vi "IR Opo Main.vi"() -> ()   [LabVIEW 2015]
uses:
  System.Windows.Forms
  D:/Fabrizio/Labview Projects/IR OPO Controller/Branches/Final version/uc480DotNet.dll
  uc480DotNet.dll
  <vilib>/Utility/miscctls.llb/LVBoundsTypeDef.ctl
  <vilib>/Utility/config.llb/Read Key (I32).vi
  OPOTEK.dll
  <vilib>/vision/NI_Vision_Development_Module.lvlib
  <vilib>/Utility/config.llb/NI_LVConfig.lvlib
panel:
  in  "Exit 4":bool
  in  "EXIT 3":bool
  in  "EXIT 2":bool
  in  "Laser spot\nX diameter":i32=250
  out "Laser Y offset":string
  out "Laser X offset":string
  in  "Laser offset \nY Position":i32=472 step=1
  in  "Laser offset \nX Position":i32=563 step=1
  out "ROI Rectangle Y position":i32
  out "ROI Rectangle X position":i32
  out "Processi time (sec)":i32
  in  "Processing time unit":string(combo)="sec"
  in  "Mode":i32(ring) items=["RGB 32"=0, "RGB 24"=1, "Y8 Monochrom"=6]
  in  "Camera":refnum<k24>(container)
  in  "Init Camera":bool
  in  "Start Live":bool
  in  "Stop Live":bool
  in  "Load Parameter":bool
  out "Error Out":errorcluster caption="error"
  out "Bits/Pixel":i32=8
  out "Width":i32=8
  out "Height":i32=8
  out "Serial Number":string
  in  "Camera ID":i32
  in  "Zoom":dbl(ring)=1.5 items=["4X"=4.0, "2X"=2.0, "1.5X"=1.5, "1.25X"=1.25, "1X"=1.0]
  in  "Gain Boost":bool=TRUE
  in  "Snapshot":bool
  out "Output":picture
  in  "Exposure":dbl(slide)=33.21525 min=0.06241666666666667 max=99.80425000000001 step=0.06241666666666667 scale=0.06241666666666667..99.80425000000001 scale format="%#.3g"
  in  "Framerate":dbl(slide)=33.21525 min=0.47411700449083627 max=15.001275108384213 step=0.014032998230479876 scale=0.47411700449083627..15.001275108384213 scale format="%#.3g"
  in  "Pixelclock":i32(slide)=33 min=5 max=40 step=1 scale=5.0..40.0
  out "Bits/Pixel 2":i32=8
  out "Width 2":i32=8
  out "Height 2":i32=8
  out "Serial Number 2":string
  in  "error in (no error)":errorcluster
  out "error out":errorcluster
  in  "Y":string="3"
  in  "X":string="2"
  out "# pixels in an ablation spot":i32=625
  in  "Sampling\nPrecision":dbl=0.8 min=0.0 max=1.0 step=0.01 format="%#_13g"
  out "Y step size in pixels":i32=12
  out "Y Step size in µm":i32=120
  out "Commands array":string[][](array[string])
  out "Laser on/off array":bool[][](array[boolean])
  out "Y axis moving time":dbl=250.0
  out "Time array":dbl[][](array[numeric])
  in  "Process Image":bool
  in  "Pixel \nsize":dbl=10.0
  in  "Axes speed \n(µm/s)":i32=500
  in  "Laser spot\nY diameter":i32=250
  in  "Y axis \nprecision":i32=2
  in  "Fast \nsampling?":bool=TRUE
  out "Y size \n(pixels)":i32
  out "X size\n(pixels)":i32
  out "Process time":dbl
  out "X size \n(µm)":i32
  out "Y size \n(µm)":i32
  out "Source":T1(plugin-control)
  in  "Delay":dbl format="%#_13g"
  in  "GPIB Mode":i16
  in  "Open ESP \nManual":bool
  in  "Type a command":string
  in  "Send \nCommand":bool
  out "GPIBtimeout":i32
  out "GPIBtermChar":i32
  out "GPIBport":i32
  out "GPIBdelay":i32
  in  "Run Program":bool
  in  "Capture":bool
  out "Log":string
  in  "Check \nProgram":bool
  out "Laser Operation":bool
  out "Current Wavelength":dbl
  in  "Alignment \ndiode":bool
  in  "LASER":bool
  in  "LAMP":bool
  in  "Wavelength":dbl min=2600.0 max=3200.0 step=1.0
  in  "TUNE":bool
  out "error_Code 3":i32
  in  "Repetition \nRate":enum16{"1", "2", "5", "10", "20"}(ring)=enum."20"
  in  "Energy (%)":i16(slide) min=0 max=100 scale=0.0..100.0 scale format="%#.1f"
  out "error_Code 2":i32
  out "Max":dbl
  out "Min":dbl
  out "error_Code":i32
  out "laserCOMPort":i32
  out "motorCOMPort":i32
  in  "EXIT":bool
  # "Laser Control"
  # "Stages Control"
  # "Camera Control"
  # "ROI Processing"
  # "Axis \nChannels"
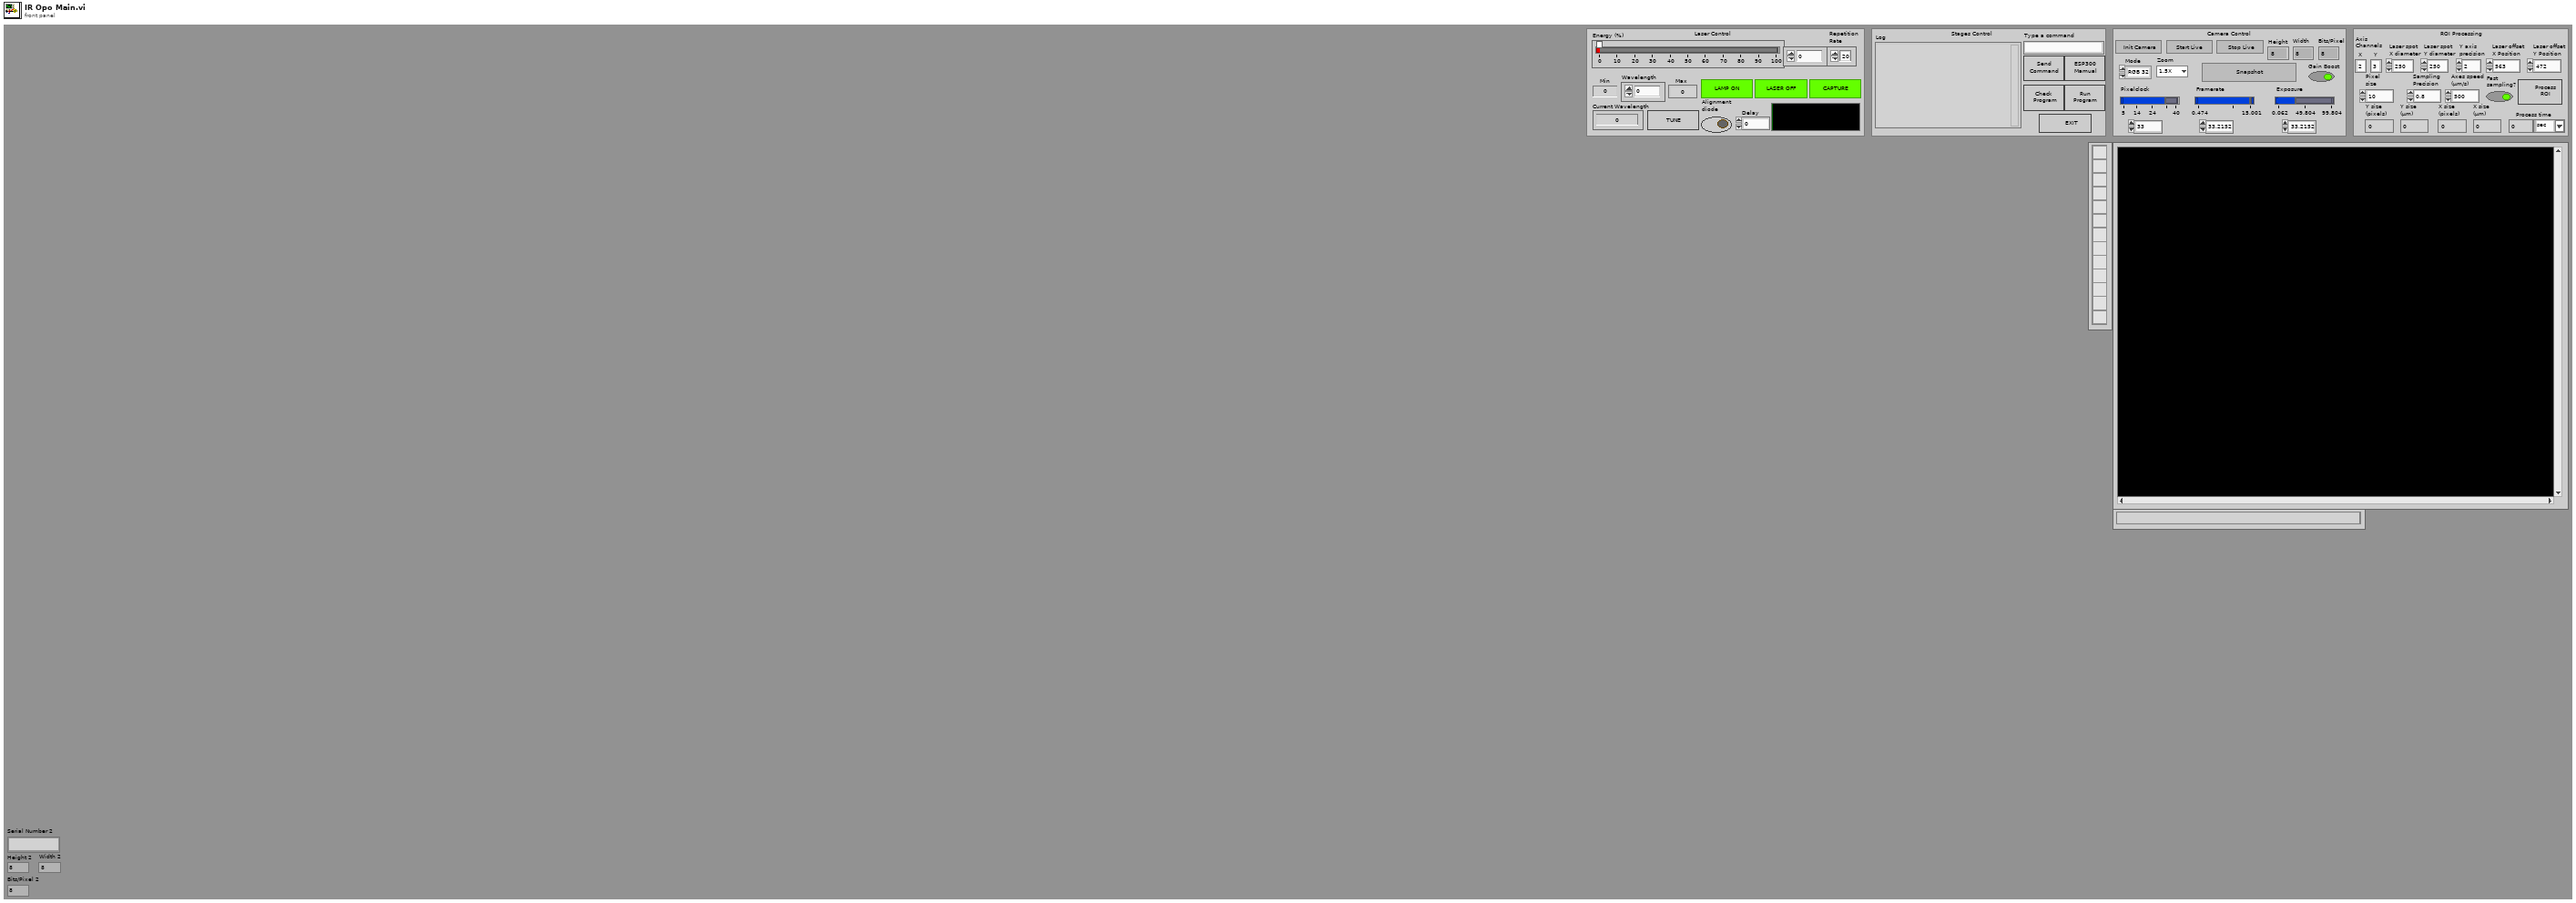
[diagram p1: front panel]
types:
  T1 = typedef "IMAQ Image.ctl" = refnum<image>
  T2 = typedef "LVBoundsTypeDef.ctl" = cluster{"Width":u32, "Height":u32}
  T3 = enum8{"Enabled", "Disabled", "Disabled and Grayed Out"}
  T4 = typedef "NI_LVConfig.lvlib/Config Data RefNum.ctl" = refnum<k1>
  T5 = typedef "Image Type" = u32
  T6 = cluster{"Global Rectangle":i32[], "Contours":cluster{"Contour Type":u32, "ROI Type":u32, "Points":i32[]}[]}
  T7 = enum16{"Initialize", "Lamp ON", "Lamp OFF", "Q-switch ON", "Q-switch OFF", "Adjust Energy", "Change Rep. Rate", "Send String"}
  T8 = enum16{"open", "replace", "create", "open or create", "replace or create", "replace or create with confirmation"}
  T9 = enum32{"invalid app kind", "Development System", "Run Time System", "Student Edition", "Embedded LabVIEW", "Evaluation", "Custom"}
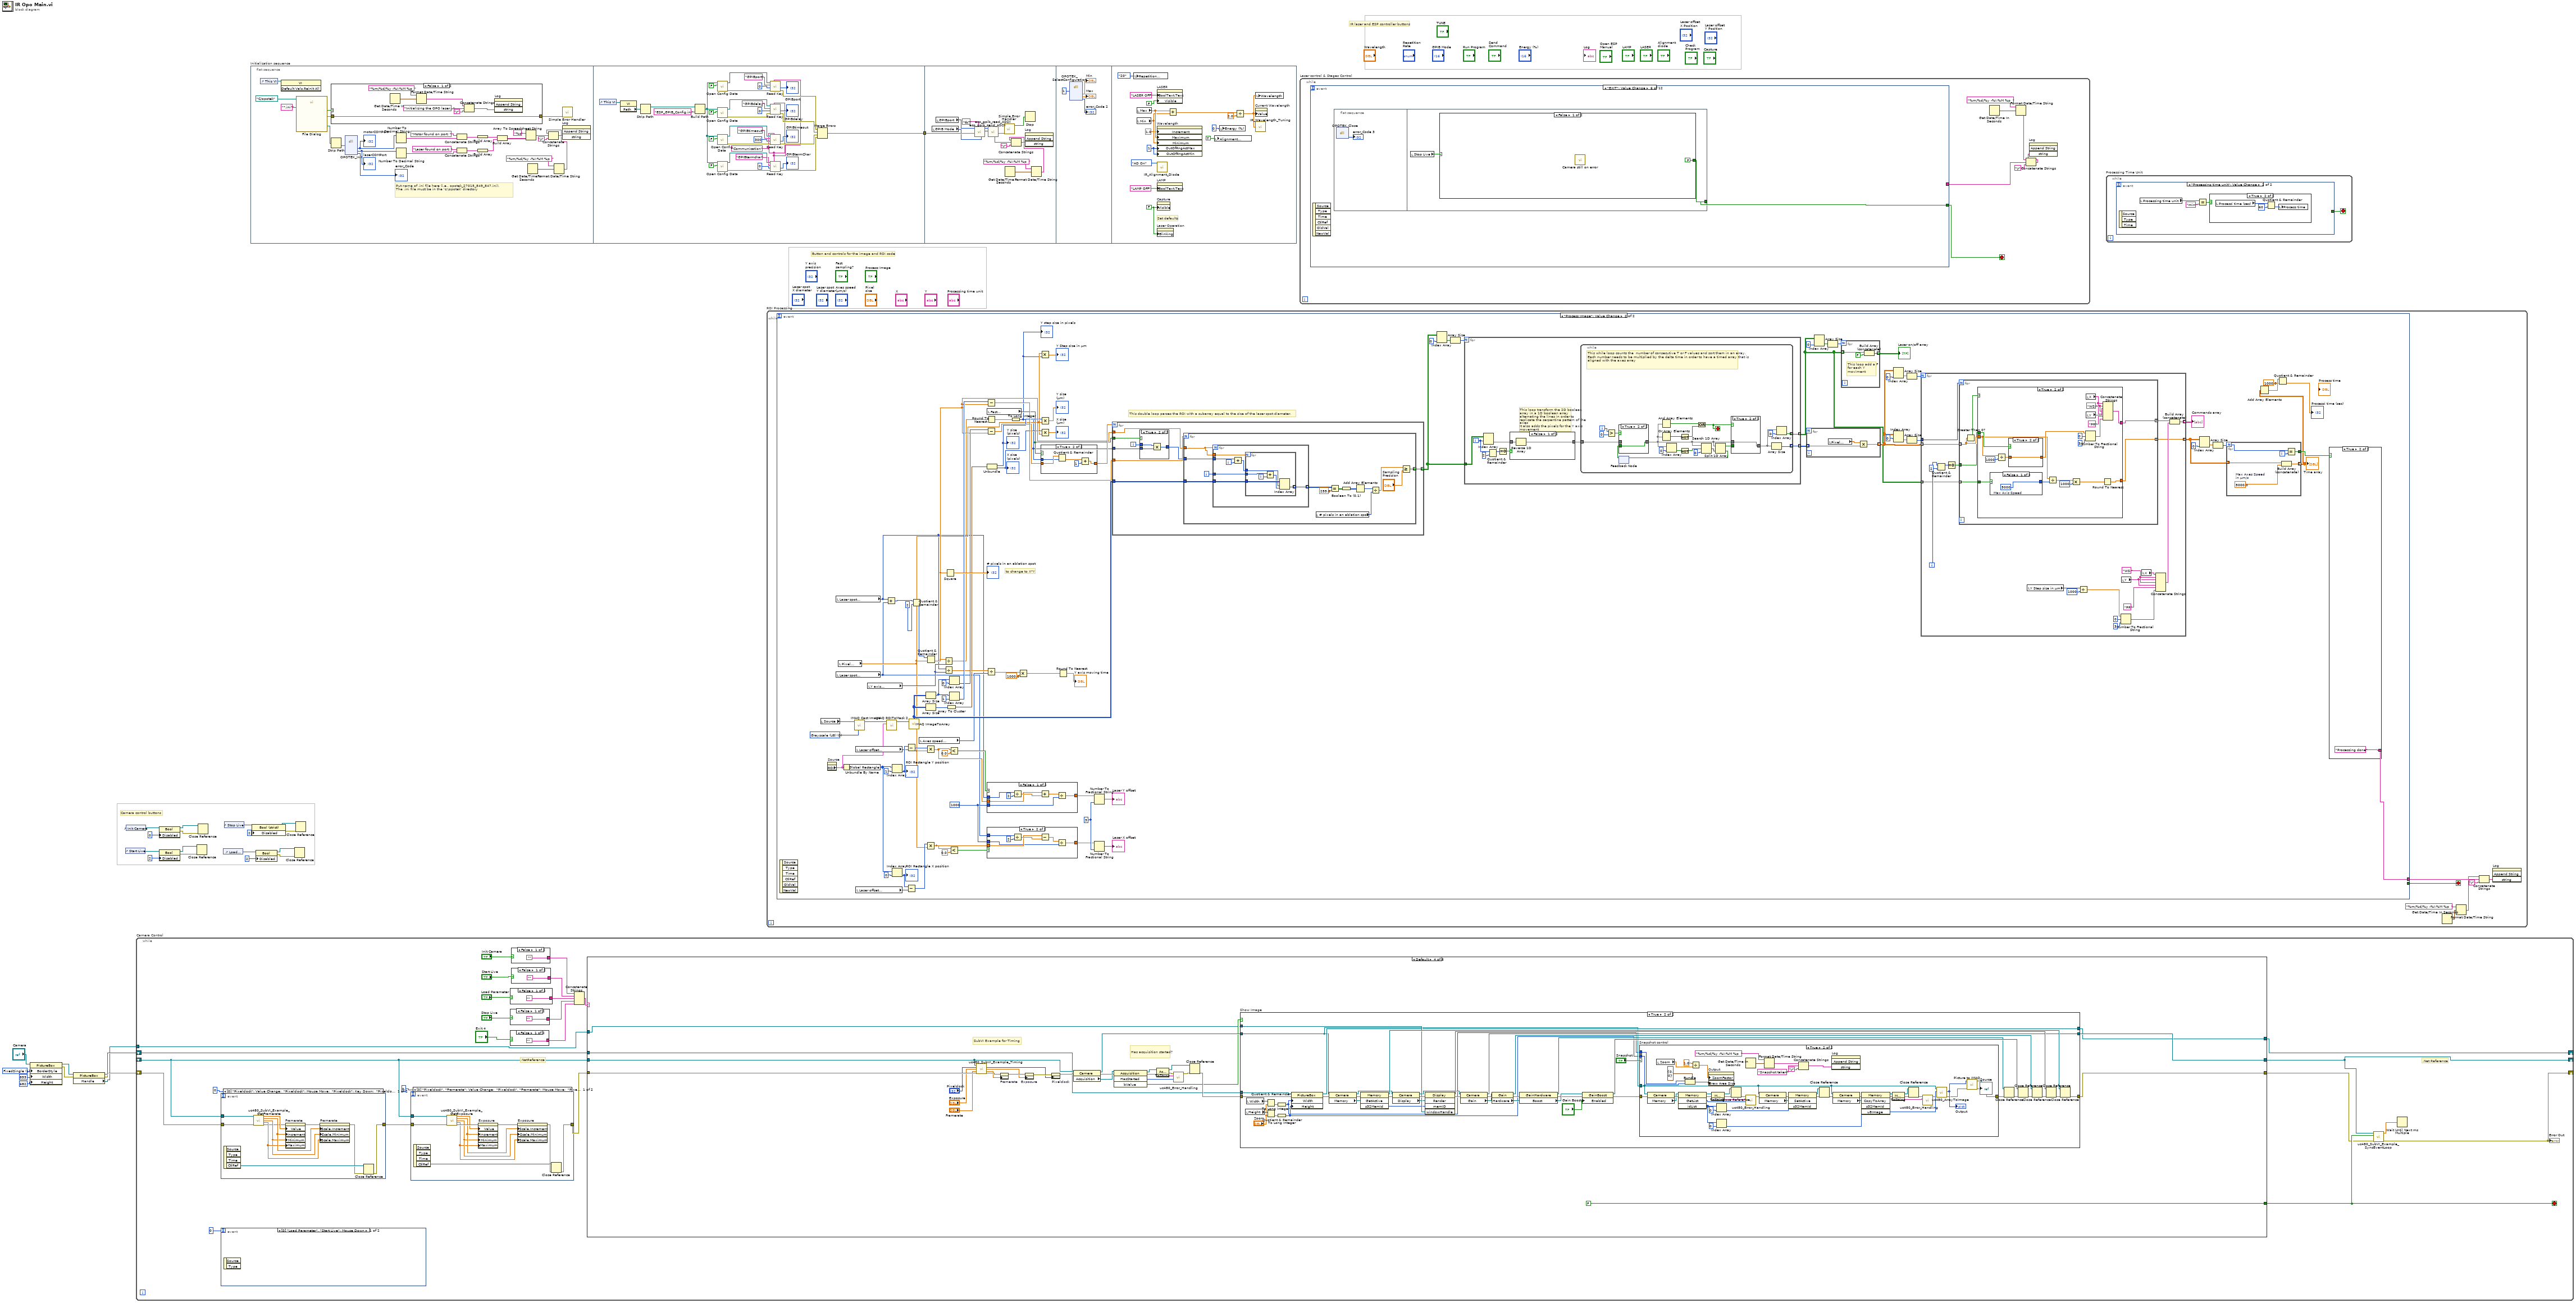
[diagram p0: block diagram]
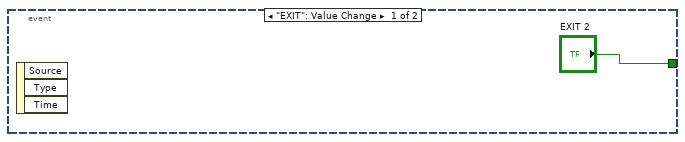
[diagram p2: hidden frame]
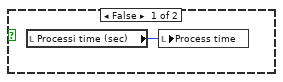
[diagram p3: hidden frame]
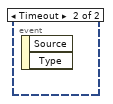
[diagram p4: hidden frame]
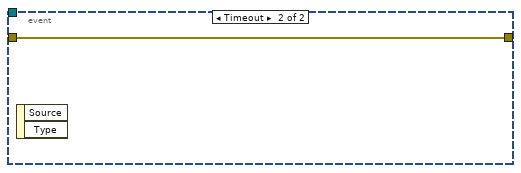
[diagram p5: hidden frame]
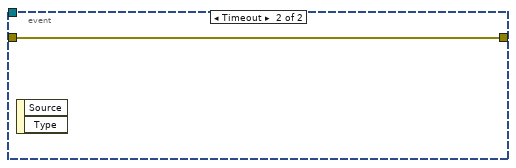
[diagram p6: hidden frame]
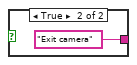
[diagram p7: hidden frame]
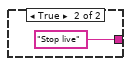
[diagram p8: hidden frame]
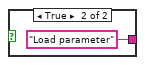
[diagram p9: hidden frame]
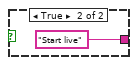
[diagram p10: hidden frame]
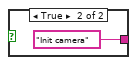
[diagram p11: hidden frame]
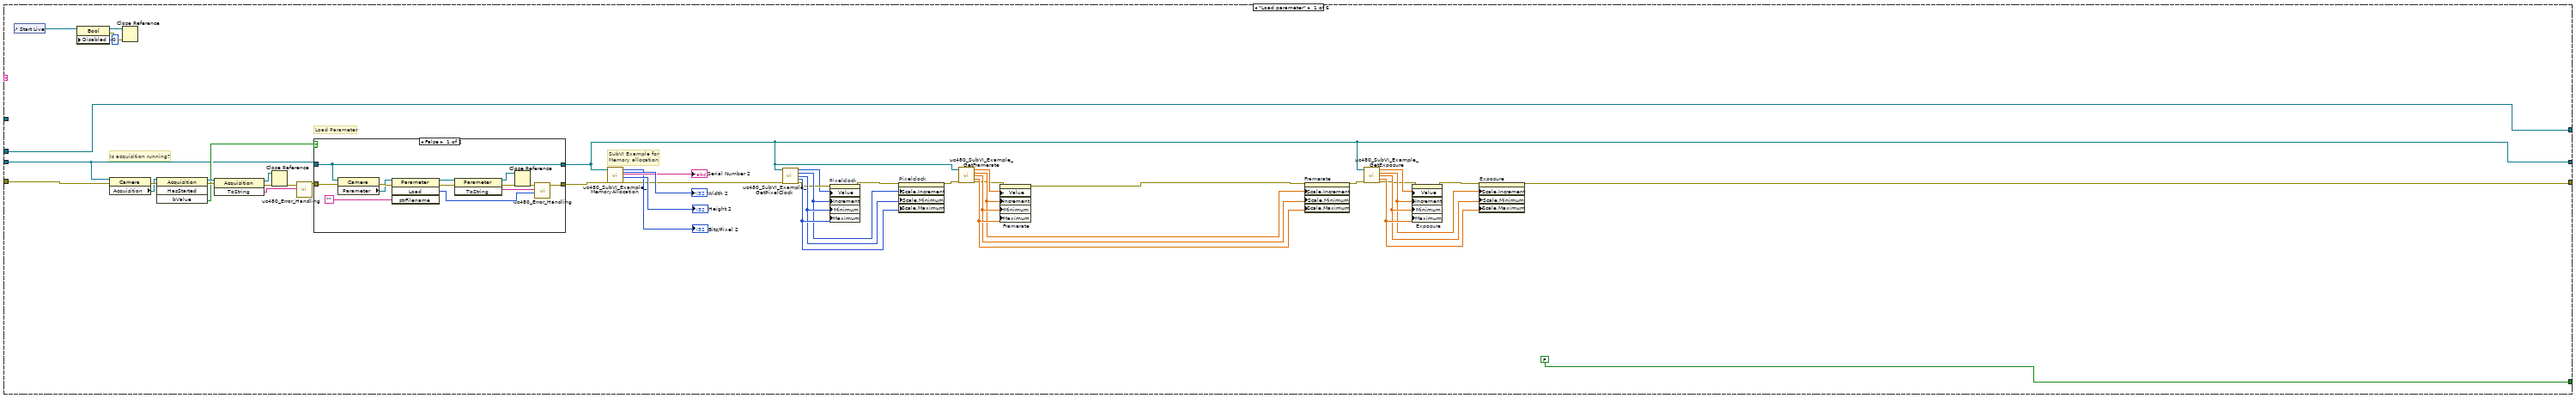
[diagram p12: hidden frame]
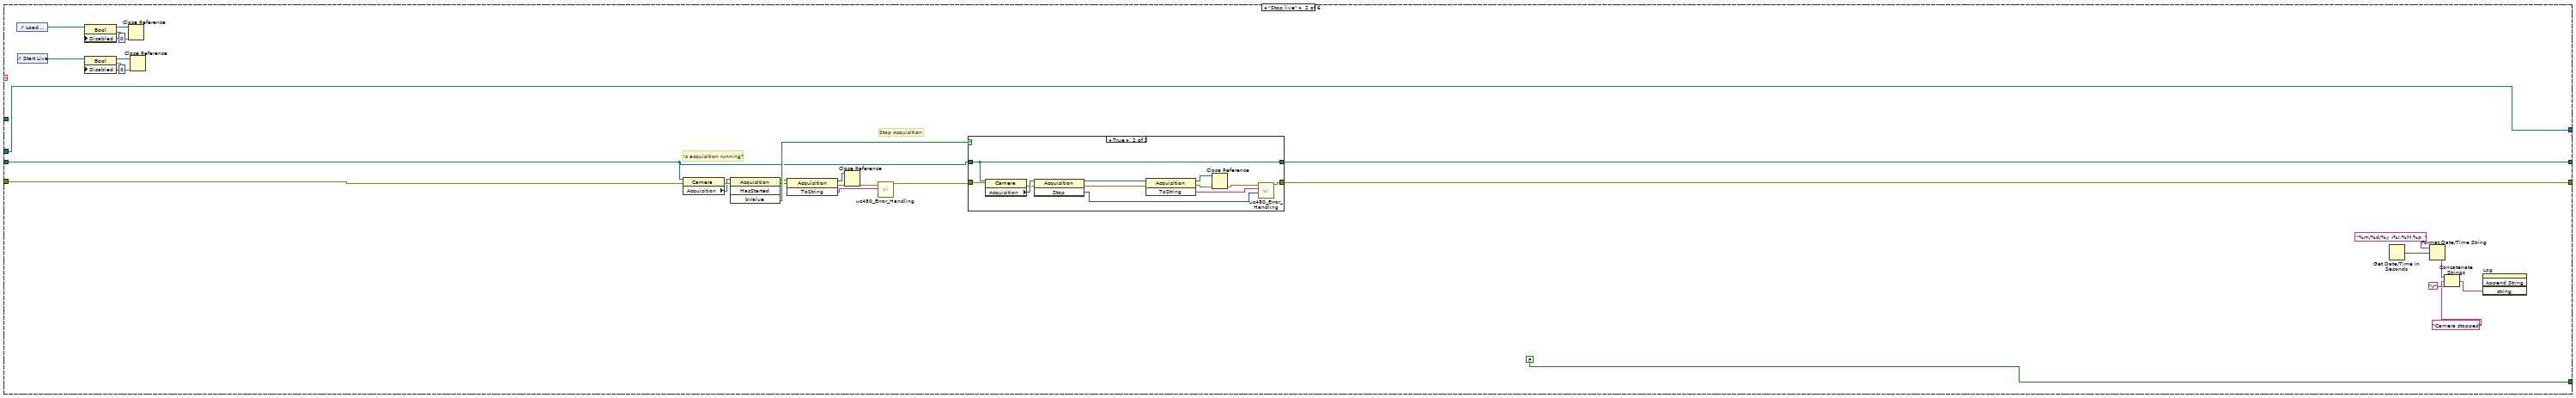
[diagram p14: hidden frame]
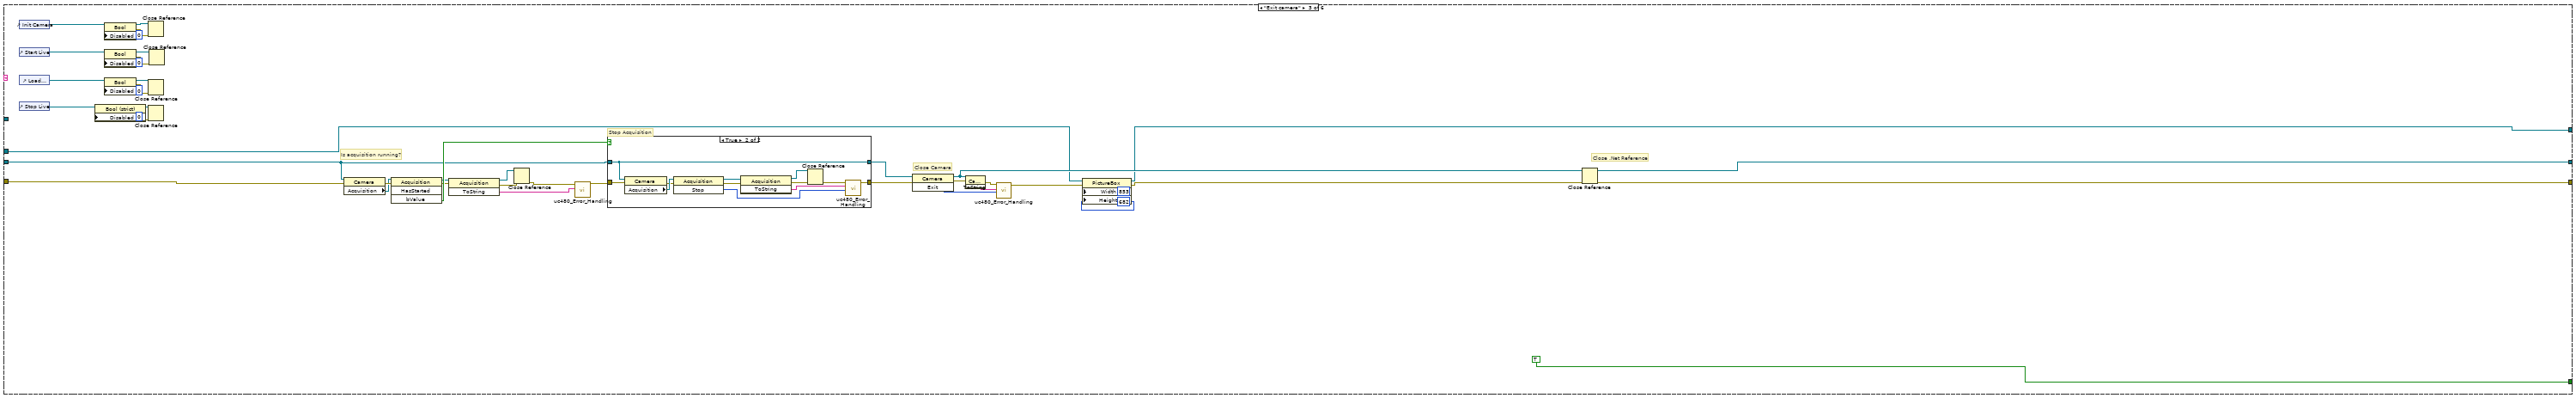
[diagram p16: hidden frame]
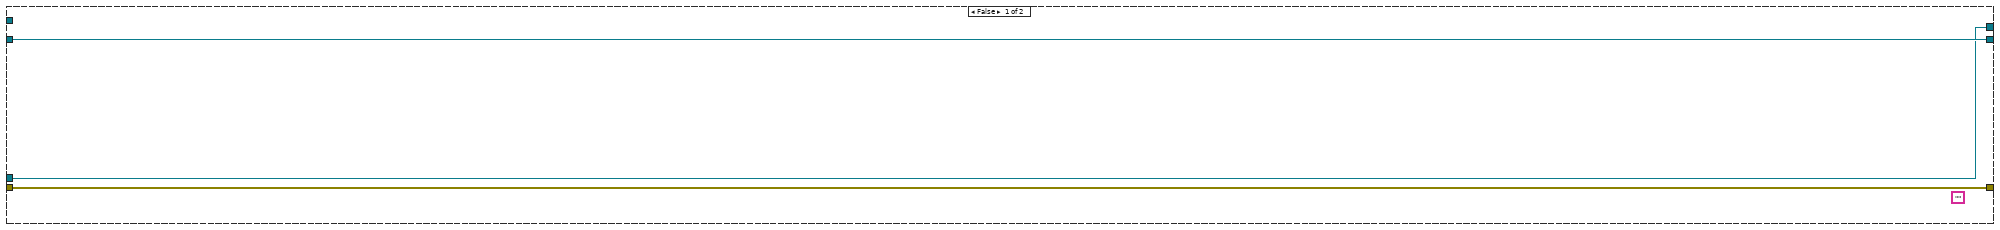
[diagram p18: hidden frame]
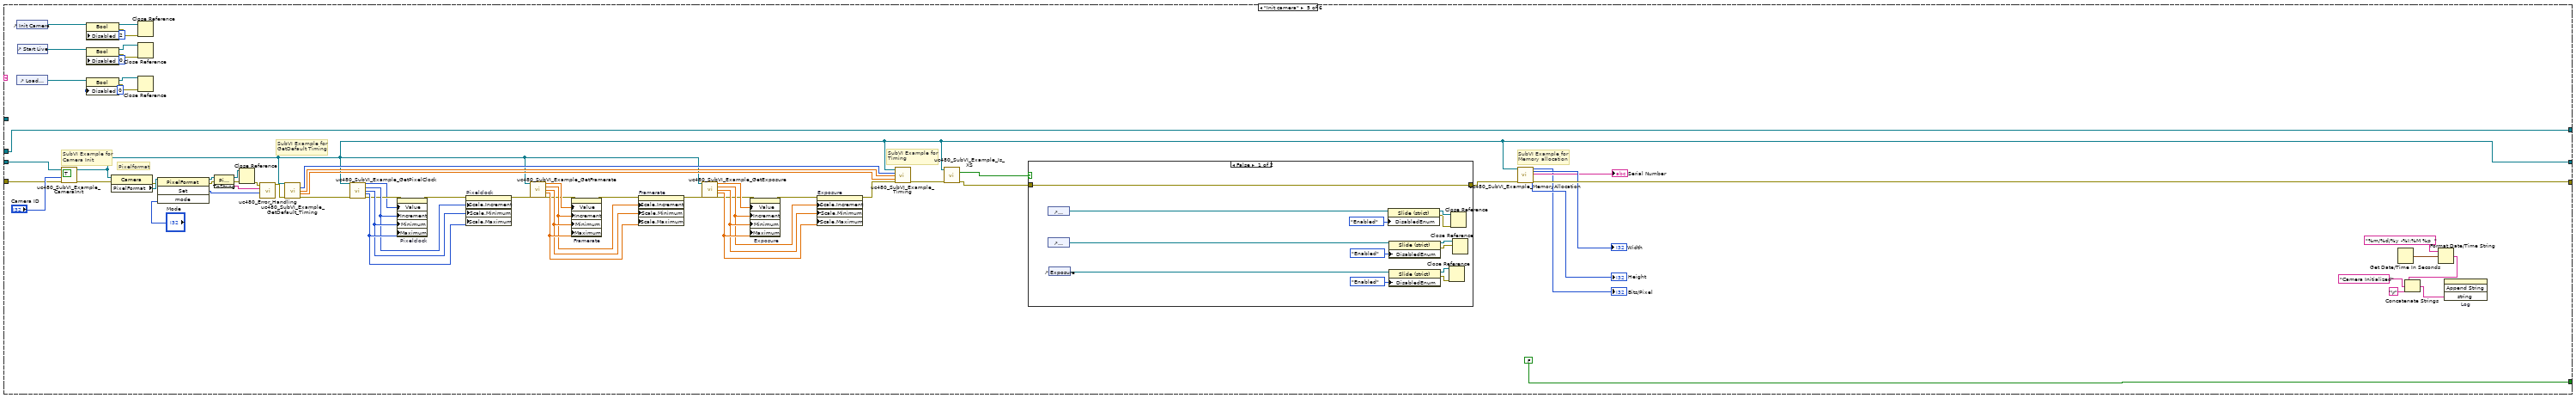
[diagram p20: hidden frame]
diagram:
  w16 = 1 items=["None", "FixedSingle", "Fixed3D"] ("BorderStyle")
  # "Camera control buttons"
  # "IR laser and ESP controller buttons"
  # "Button and controls for the image and ROI code"
  n1 = property class="PictureBox"(reference="Camera", "BorderStyle"=w16, "Width"=853, "Height"=682) -> (reference out=w4:refnum<k24>, error out=w5:errorcluster)  [unwired: 1 in]
  n2 = property class="PictureBox"(reference=w4, error in=w5) -> (reference out=w3:refnum<k24>, error out=w2:errorcluster, "Handle"=w1:refnum<k24>)
  n3 = control-ref of="Start Live"() -> (w22:refnum<vi>)
  n4 = control-ref of="Init Camera"() -> (w25:refnum<vi>)
  n5 = while "Camera Control" {
    shift-right: [w32] -> _
    shift-left: w2 -> [w38]
    shift-right: [w35] -> _
    shift-left: _ -> [w28]
    shift-right: [w30] -> _
    shift-left: w3 -> [w31]
    tunnel: w1 -> [w29]
    stop <- w36 stop-if-true
    # ".NetReference"
    # ".Net Reference"
    n6 = event shown="[0] \"Pixelclock\": Value Change;  \"Pixelclock\": Mouse Move;  \"Pixelclock\": Key Down;  \"Pixelclock\": Mouse Up" {
      selector: _ -> [_ _]
      dyn-events: _ -> [_ _]
      timeout: 0 -> [_ _]
      tunnel: [w53 w64] -> w39
      tunnel: w38 -> [w63 w64]
      tunnel: w28 -> [w62 _]
      event "Pixelclock": Value Change; "Pixelclock": Mouse Move; "Pixelclock": Key Down; "Pixelclock": Mouse Up {
        n7 = event-data() -> ("CtlRef"=w55:refnum<vi>)  [unwired: 1 in, 3 out]
        n8 = call "uc480_SubVI_Example_GetFramerate.vi"(".NET (Reference)"=w62, "Error In"=w63) -> ("Framerate"=w61:dbl, "Inc"=w60:dbl, "Min"=w58:dbl, "Max"=w59:dbl, "error out"=w57:errorcluster)  [unwired: 9 in]
        n9 = property on="Framerate" class="Slide (strict)"(error in=w57, "Value"=w61, "Increment"=w60, "Minimum"=w58, "Maximum"=w59) -> (error out=w56:errorcluster)  [unwired: 1 in, 1 out]
        n10 = property on="Framerate" class="Slide (strict)"(error in=w56, "Scale.Increment"=w60, "Scale.Minimum"=w58, "Scale.Maximum"=w59) -> (error out=w54:errorcluster)  [unwired: 1 in, 1 out]
        n11 = Close Reference(reference=w55, error in (no error)=w54) -> (error out=w53:errorcluster)
      }
      event Timeout {
        n12 = event-data() -> ()  [unwired: 1 in, 2 out]
      }
    }
    n13 = event shown="[0] \"Load Parameter\", \"Start Live\": Mouse Down" {
      selector: _ -> [_ _]
      dyn-events: _ -> [_ _]
      timeout: 0 -> [_ _]
      event "Load Parameter", "Start Live": Mouse Down {
        n14 = event-data() -> ()  [unwired: 1 in, 2 out]
      }
      event Timeout {
        n15 = event-data() -> ()  [unwired: 1 in, 2 out]
      }
    }
    n16 = event shown="[0] \"Pixelclock\", \"Framerate\": Value Change;  \"Pixelclock\", \"Framerate\": Mouse Move;  \"Pixelclock\", \"Framerate\": Key Down;  \"Pixelclock\", \"Framerate\": Mouse Up" {
      selector: _ -> [_ _]
      dyn-events: _ -> [_ _]
      timeout: 0 -> [_ _]
      tunnel: w39 -> [w75 w76]
      tunnel: [w65 w76] -> w41
      tunnel: w28 -> [w74 _]
      event "Pixelclock", "Framerate": Value Change; "Pixelclock", "Framerate": Mouse Move; "Pixelclock", "Framerate": Key Down; "Pixelclock", "Framerate": Mouse Up {
        n17 = event-data() -> ("CtlRef"=w67:refnum<vi>)  [unwired: 1 in, 3 out]
        n18 = call "uc480_SubVI_Example_GetExposure.vi"(".NET (Reference)"=w74, "Error In"=w75) -> ("Exposure"=w71:dbl, "Inc"=w70:dbl, "Min"=w69:dbl, "Max"=w68:dbl, "Error out"=w72:errorcluster)  [unwired: 9 in]
        n19 = property on="Exposure" class="Slide (strict)"(error in=w72, "Value"=w71, "Increment"=w70, "Minimum"=w69, "Maximum"=w68) -> (error out=w73:errorcluster)  [unwired: 1 in, 1 out]
        n20 = property on="Exposure" class="Slide (strict)"(error in=w73, "Scale.Increment"=w70, "Scale.Minimum"=w69, "Scale.Maximum"=w68) -> (error out=w66:errorcluster)  [unwired: 1 in, 1 out]
        n21 = Close Reference(reference=w67, error in (no error)=w66) -> (error out=w65:errorcluster)
      }
      event Timeout {
        n22 = event-data() -> ()  [unwired: 1 in, 2 out]
      }
    }
    n23 = case shown="False" "Exit 4" {
      tunnel: ["" "Exit camera"] -> w43
      frame False {
      }
      frame True {
      }
    }
    n24 = case shown="False" "Load Parameter" {
      tunnel: ["" "Load parameter"] -> w46
      frame False {
      }
      frame True {
      }
    }
    n25 = case shown="False" "Stop Live" {
      tunnel: ["" "Stop live"] -> w45
      frame False {
      }
      frame True {
      }
    }
    n26 = case shown="False" "Init Camera" {
      tunnel: ["" "Init camera"] -> w50
      frame False {
      }
      frame True {
      }
    }
    n27 = case shown="False" "Start Live" {
      tunnel: ["" "Start live"] -> w49
      frame False {
      }
      frame True {
      }
    }
    n28 = Concatenate Strings(w50, w49, w46, w45, w43) -> (w48:string)
    n29 = case shown="Default" w48 {
      tunnel: w28 -> [w123 w169 w219 w261 w437 w494]
      tunnel: w41 -> [w126 w170 w220 w271 w436 w495]
      tunnel: [w93 w168 w228 w270 w395 w493] -> w35
      tunnel: [w94 w167 w229 w269 w432 w491] -> w34
      tunnel: [FALSE FALSE TRUE FALSE FALSE FALSE] -> w36
      tunnel: w31 -> [w92 w161 w201 w253 w390 w484]
      tunnel: [w92 w161 w200 w252 w390 w484] -> w30
      tunnel: w29 -> [_ _ _ w249 _ _]
      frame "Load parameter" {
        # "SubVI Example for \nMemory allocation"
        # "Is acquisition running?"
        # "Load Parameter"
        n30 = control-ref of="Start Live"() -> (w117:refnum<vi>)
        n31 = property class="Bool"(reference=w117, "Disabled"=u8 0 ("Deaktiviert")) -> (reference out=w91:refnum<vi>, error out=w90:errorcluster)  [unwired: 1 in]
        n32 = property class="Camera"(reference=w123, error in=w126) -> (error out=w131:errorcluster, "Acquisition"=w130:refnum<k24>)  [unwired: 1 out]
        n33 = Close Reference(reference=w91, error in (no error)=w90) -> ()  [unwired: 1 out]
        n34 = invoke class="Acquisition" method="HasStarted"(reference=w130, error in=w131) -> (reference out=w127:refnum<k24>, error out=w129:errorcluster, "bValue"=w125:bool)  [unwired: 2 in, 1 out]
        n35 = invoke class="Acquisition" method="ToString"(reference=w127, error in=w129) -> (reference out=w89:refnum<k24>, error out=w88:errorcluster, "ToString"=w128:string)  [unwired: 1 in]
        n36 = Close Reference(reference=w89, error in (no error)=w88) -> (error out=w87:errorcluster)
        n37 = call "uc480_Error_Handling.vi"("Error String"=w128, "Error In"=w87) -> ("Error Out"=w124:errorcluster)  [unwired: 9 in]
        n38 = case shown="False" w125 {
          tunnel: w124 -> [w139 w146]
          tunnel: w123 -> [w137 w147]
          tunnel: [w138 w146] -> w118
          tunnel: [w137 w147] -> w93
          frame False {
            n39 = property class="Camera"(reference=w137, error in=w139) -> (error out=w141:errorcluster, "Parameter"=w140:refnum<k24>)  [unwired: 1 out]
            n40 = invoke class="Parameter" method="Load"(reference=w140, error in=w141, "strFilename"="") -> (reference out=w143:refnum<k24>, error out=w144:errorcluster, "Load"=w136:i32)  [unwired: 1 in, 1 out]
            n41 = invoke class="Parameter" method="ToString"(reference=w143, error in=w144) -> (reference out=w133:refnum<k24>, error out=w135:errorcluster, "ToString"=w145:string)  [unwired: 1 in]
            n42 = Close Reference(reference=w133, error in (no error)=w135) -> (error out=w134:errorcluster)
            n43 = call "uc480_Error_Handling.vi"("Error Code"=w136, "Error String"=w145, "Error In"=w134) -> ("Error Out"=w138:errorcluster)  [unwired: 8 in]
          }
          frame True {
          }
        }
        n44 = call "uc480_SubVI_Example_MemoryAllocation.vi"(".NET (Reference)"=w93, "Error In"=w118) -> ("Bits/Pixel 2"=→"Bits/Pixel 2":i32, "Width"=→"Width 2":i32, "Serial Number"=→"Serial Number 2":string, "Height"=→"Height 2":i32, "Error Out"=w95:errorcluster)  [unwired: 13 in]
        n45 = call "uc480_SubVI_Example_GetPixelClock.vi"(".NET (Reference)"=w93, "Error In"=w95) -> ("Pixel Clock"=w96:i32, "Inc"=w98:i32, "Min"=w99:i32, "Max"=w100:i32, "error out"=w97:errorcluster)  [unwired: 9 in]
        n46 = property on="Pixelclock" class="Slide (strict)"(error in=w97, "Value"=w96, "Increment"=w98, "Minimum"=w99, "Maximum"=w100) -> (error out=w101:errorcluster)  [unwired: 1 in, 1 out]
        n47 = property on="Pixelclock" class="Slide (strict)"(error in=w101, "Scale.Increment"=w98, "Scale.Minimum"=w99, "Scale.Maximum"=w100) -> (error out=w102:errorcluster)  [unwired: 1 in, 1 out]
        n48 = call "uc480_SubVI_Example_GetFramerate.vi"(".NET (Reference)"=w93, "Error In"=w102) -> ("Framerate"=w105:dbl, "Inc"=w106:dbl, "Min"=w107:dbl, "Max"=w108:dbl, "error out"=w104:errorcluster)  [unwired: 9 in]
        n49 = property on="Framerate" class="Slide (strict)"(error in=w104, "Value"=w105, "Increment"=w106, "Minimum"=w107, "Maximum"=w108) -> (error out=w103:errorcluster)  [unwired: 1 in, 1 out]
        n50 = property on="Framerate" class="Slide (strict)"(error in=w103, "Scale.Increment"=w106, "Scale.Minimum"=w107, "Scale.Maximum"=w108) -> (error out=w109:errorcluster)  [unwired: 1 in, 1 out]
        n51 = call "uc480_SubVI_Example_GetExposure.vi"(".NET (Reference)"=w93, "Error In"=w109) -> ("Exposure"=w112:dbl, "Inc"=w113:dbl, "Min"=w114:dbl, "Max"=w115:dbl, "Error out"=w110:errorcluster)  [unwired: 9 in]
        n52 = property on="Exposure" class="Slide (strict)"(error in=w110, "Value"=w112, "Increment"=w113, "Minimum"=w114, "Maximum"=w115) -> (error out=w111:errorcluster)  [unwired: 1 in, 1 out]
        n53 = property on="Exposure" class="Slide (strict)"(error in=w111, "Scale.Increment"=w113, "Scale.Minimum"=w114, "Scale.Maximum"=w115) -> (error out=w94:errorcluster)  [unwired: 1 in, 1 out]
      }
      frame "Stop live" {
        # "Is acquisition running?"
        # "Stop Acquisition"
        n54 = control-ref of="Load Parameter"() -> (w165:refnum<vi>)
        n55 = control-ref of="Start Live"() -> (w162:refnum<vi>)
        n56 = property class="Bool"(reference=w165, "Disabled"=u8 0 ("Deaktiviert")) -> (reference out=w160:refnum<vi>, error out=w159:errorcluster)  [unwired: 1 in]
        n57 = property class="Bool"(reference=w162, "Disabled"=u8 0 ("Deaktiviert")) -> (reference out=w158:refnum<vi>, error out=w157:errorcluster)  [unwired: 1 in]
        n58 = Close Reference(reference=w160, error in (no error)=w159) -> ()  [unwired: 1 out]
        n59 = Close Reference(reference=w158, error in (no error)=w157) -> ()  [unwired: 1 out]
        n60 = property class="Camera"(reference=w169, error in=w170) -> (error out=w177:errorcluster, "Acquisition"=w176:refnum<k24>)  [unwired: 1 out]
        n61 = invoke class="Acquisition" method="HasStarted"(reference=w176, error in=w177) -> (reference out=w171:refnum<k24>, error out=w173:errorcluster, "bValue"=w175:bool)  [unwired: 2 in, 1 out]
        n62 = invoke class="Acquisition" method="ToString"(reference=w171, error in=w173) -> (reference out=w154:refnum<k24>, error out=w156:errorcluster, "ToString"=w172:string)  [unwired: 1 in]
        n63 = Close Reference(reference=w154, error in (no error)=w156) -> (error out=w155:errorcluster)
        n64 = call "uc480_Error_Handling.vi"("Error String"=w172, "Error In"=w155) -> ("Error Out"=w174:errorcluster)  [unwired: 9 in]
        n65 = case shown="True" w175 {
          tunnel: [w179 w190] -> w167
          tunnel: w174 -> [w179 w191]
          tunnel: w169 -> [w178 w183]
          tunnel: [w178 w183] -> w168
          frame False {
          }
          frame True {
            n66 = property class="Camera"(reference=w183, error in=w191) -> (error out=w187:errorcluster, "Acquisition"=w188:refnum<k24>)  [unwired: 1 out]
            n67 = invoke class="Acquisition" method="Stop"(reference=w188, error in=w187) -> (reference out=w185:refnum<k24>, error out=w186:errorcluster, "Stop"=w184:i32)  [unwired: 1 in]
            n68 = invoke class="Acquisition" method="ToString"(reference=w185, error in=w186) -> (reference out=w180:refnum<k24>, error out=w182:errorcluster, "ToString"=w189:string)  [unwired: 1 in]
            n69 = Close Reference(reference=w180, error in (no error)=w182) -> (error out=w181:errorcluster)
            n70 = call "uc480_Error_Handling.vi"("Error Code"=w184, "Error String"=w189, "Error In"=w181) -> ("Error Out"=w190:errorcluster)  [unwired: 8 in]
          }
        }
        n71 = Get Date/Time In Seconds() -> (seconds since 1Jan1904=w149:timestamp)
        n72 = Format Date/Time String(time format string (%c)="%m/%d/%y -%I:%M %p  ", seconds (now)=w149) -> (date/time string=w148:string)  [unwired: 1 in]
        n73 = Concatenate Strings(w148, "Camera stopped", "\r") -> (w153:string)
        n74 = invoke on="Log" class="Str" method="Append String"("string"=w153) -> ()  [unwired: 3 in, 4 out]
      }
      frame "Exit camera" {
        # "Close .Net Reference"
        # "Is acquisition running?"
        # "Stop Acquisition"
        # "Close Camera"
        n75 = control-ref of="Init Camera"() -> (w212:refnum<vi>)
        n76 = control-ref of="Start Live"() -> (w211:refnum<vi>)
        n77 = control-ref of="Load Parameter"() -> (w210:refnum<vi>)
        n78 = control-ref of="Stop Live"() -> (w209:refnum<vi>)
        n79 = property class="Bool (strict)"(reference=w209, "Disabled"=u8 0 ("Deaktiviert")) -> (reference out=w199:refnum<vi>, error out=w198:errorcluster)  [unwired: 1 in]
        n80 = property class="Bool"(reference=w212, "Disabled"=u8 0 ("Deaktiviert")) -> (reference out=w193:refnum<vi>, error out=w192:errorcluster)  [unwired: 1 in]
        n81 = property class="Bool"(reference=w211, "Disabled"=u8 0 ("Deaktiviert")) -> (reference out=w195:refnum<vi>, error out=w194:errorcluster)  [unwired: 1 in]
        n82 = property class="Bool"(reference=w210, "Disabled"=u8 0 ("Deaktiviert")) -> (reference out=w197:refnum<vi>, error out=w196:errorcluster)  [unwired: 1 in]
        n83 = Close Reference(reference=w193, error in (no error)=w192) -> ()  [unwired: 1 out]
        n84 = Close Reference(reference=w197, error in (no error)=w196) -> ()  [unwired: 1 out]
        n85 = Close Reference(reference=w199, error in (no error)=w198) -> ()  [unwired: 1 out]
        n86 = Close Reference(reference=w195, error in (no error)=w194) -> ()  [unwired: 1 out]
        n87 = property class="Camera"(reference=w219, error in=w220) -> (error out=w227:errorcluster, "Acquisition"=w226:refnum<k24>)  [unwired: 1 out]
        n88 = invoke class="Acquisition" method="HasStarted"(reference=w226, error in=w227) -> (reference out=w221:refnum<k24>, error out=w223:errorcluster, "bValue"=w225:bool)  [unwired: 2 in, 1 out]
        n89 = invoke class="Acquisition" method="ToString"(reference=w221, error in=w223) -> (reference out=w206:refnum<k24>, error out=w208:errorcluster, "ToString"=w222:string)  [unwired: 1 in]
        n90 = Close Reference ("Close Referenz")(reference=w206, error in (no error)=w208) -> (error out=w207:errorcluster)
        n91 = call "uc480_Error_Handling.vi"("Error String"=w222, "Error In"=w207) -> ("Error Out"=w224:errorcluster)  [unwired: 9 in]
        n92 = case shown="True" w225 {
          tunnel: [w236 w247] -> w217
          tunnel: w224 -> [w236 w248]
          tunnel: w219 -> [w235 w240]
          tunnel: [w235 w240] -> w218
          frame False {
          }
          frame True {
            n93 = property class="Camera"(reference=w240, error in=w248) -> (error out=w244:errorcluster, "Acquisition"=w245:refnum<k24>)  [unwired: 1 out]
            n94 = invoke class="Acquisition" method="Stop"(reference=w245, error in=w244) -> (reference out=w242:refnum<k24>, error out=w243:errorcluster, "Stop"=w241:i32)  [unwired: 1 in]
            n95 = invoke class="Acquisition" method="ToString"(reference=w242, error in=w243) -> (reference out=w237:refnum<k24>, error out=w239:errorcluster, "ToString"=w246:string)  [unwired: 1 in]
            n96 = Close Reference ("Close Referenz")(reference=w237, error in (no error)=w239) -> (error out=w238:errorcluster)
            n97 = call "uc480_Error_Handling.vi"("Error Code"=w241, "Error String"=w246, "Error In"=w238) -> ("Error Out"=w247:errorcluster)  [unwired: 8 in]
          }
        }
        n98 = invoke class="Camera" method="Exit"(reference=w218, error in=w217) -> (reference out=w228:refnum<k24>, error out=w231:errorcluster, "Exit"=w230:i32)  [unwired: 1 in]
        n99 = invoke class="Camera" method="ToString"(reference=w228, error in=w231) -> (error out=w232:errorcluster, "ToString"=w233:string)  [unwired: 1 in, 1 out]
        n100 = call "uc480_Error_Handling.vi"("Error Code"=w230, "Error String"=w233, "Error In"=w232) -> ("Error Out"=w205:errorcluster)  [unwired: 8 in]
        n101 = property class="PictureBox"(reference=w201, error in=w205, "Width"=853, "Height"=682) -> (reference out=w200:refnum<k24>, error out=w204:errorcluster)
        n102 = Close Reference ("Close Referenz")(reference=w228, error in (no error)=w204) -> (error out=w229:errorcluster)
      }
      frame Default {
        # "SubVI Example for Timing"
        # "Has acquisition started?"
        n103 = call "uc480_SubVI_Example_Timing.vi"(".NET (Reference)"=w261, "Pixelclock"="Pixelclock", "Exposure time"="Exposure", "Framerate"="Framerate", "Error In"=w271) -> ("Pixelclock"=w264:i32, "Exposure time"=w263:dbl, "Framerate"=w262:dbl, "Error Out"=w268:errorcluster)  [unwired: 7 in]
        n104 = property on="Framerate" class="Schieber (strikt)"(error in=w268, "Scale.RngStart"=w262) -> (error out=w267:errorcluster)  [unwired: 1 in, 1 out]
        n105 = property on="Exposure" class="Schieber (strikt)"(error in=w267, "Scale.RngStart"=w263) -> (error out=w266:errorcluster)  [unwired: 1 in, 1 out]
        n106 = property on="Pixelclock" class="Schieber (strikt)"(error in=w266, "Scale.RngStart"=w264) -> (error out=w265:errorcluster)  [unwired: 1 in, 1 out]
        n107 = property class="Camera"(reference=w261, error in=w265) -> (reference out=w254:refnum<k24>, error out=w277:errorcluster, "Acquisition"=w276:refnum<k24>)
        n108 = invoke class="Acquisition" method="HasStarted"(reference=w276, error in=w277) -> (reference out=w251:refnum<k24>, error out=w273:errorcluster, "HasStarted"=w272:i32, "bValue"=w250:bool)  [unwired: 2 in]
        n109 = invoke class="Acquisition" method="ToString"(reference=w251, error in=w273) -> (reference out=w255:refnum<k24>, error out=w275:errorcluster, "ToString"=w274:string)  [unwired: 1 in]
        n110 = call "uc480_Error_Handling.vi"("Error Code"=w272, "Error String"=w274, "Error In"=w275) -> ("Error Out"=w257:errorcluster)  [unwired: 8 in]
        n111 = Close Reference(reference=w255, error in (no error)=w257) -> (error out=w256:errorcluster)
        n112 = case "Show Image" shown="True" w250 {
          tunnel: [w281 w293] -> w269
          tunnel: w256 -> [w281 w321]
          tunnel: w254 -> [w280 w285]
          tunnel: [w280 w289] -> w270
          tunnel: w253 -> [w279 w310]
          tunnel: [w279 w287] -> w252
          tunnel: w249 -> [_ w317]
          frame False {
            (unwired) ""
          }
          frame True {
            n113 = local read "Height"() -> (w314:i32)
            n114 = local read "Width"() -> (w315:i32)
            n115 = Quotient & Remainder(x=w315, y="Zoom") -> (floor(x/y)=w312:dbl)  [unwired: 1 out]
            n116 = Quotient & Remainder(x=w314, y="Zoom") -> (floor(x/y)=w311:dbl)  [unwired: 1 out]
            n117 = To Long Integer(number=w312) -> (32bit integer=w284:i32)
            n118 = To Long Integer(number=w311) -> (32bit integer=w283:i32)
            n119 = property class="PictureBox"(reference=w310, error in=w321, "Width"=w284, "Height"=w283) -> (reference out=w287:refnum<k24>, error out=w316:errorcluster)
            n120 = property class="Camera"(reference=w285, error in=w316) -> (reference out=w286:refnum<k24>, error out=w323:errorcluster, "Memory"=w324:refnum<k24>)
            n121 = invoke class="Memory" method="GetActive"(reference=w324, error in=w323) -> (reference out=w318:refnum<k24>, error out=w319:errorcluster, "s32MemId"=w290:i32)  [unwired: 2 in, 1 out]
            n122 = property class="Camera"(reference=w286, error in=w319) -> (reference out=w298:refnum<k24>, error out=w322:errorcluster, "Display"=w307:refnum<k24>)
            n123 = invoke class="Display" method="Render"(reference=w307, error in=w322, "memID"=w290, "windowHandle"=w317) -> (reference out=w308:refnum<k24>, error out=w309:errorcluster)  [unwired: 1 in, 3 out]
            n124 = property class="Camera"(reference=w298, error in=w309) -> (reference out=w289:refnum<k24>, error out=w305:errorcluster, "Gain"=w303:refnum<k24>)
            n125 = property class="Gain"(reference=w303, error in=w305) -> (reference out=w304:refnum<k24>, error out=w300:errorcluster, "Hardware"=w299:refnum<k24>)
            n126 = property class="GainHardware"(reference=w299, error in=w300) -> (reference out=w296:refnum<k24>, error out=w301:errorcluster, "Boost"=w302:refnum<k24>)
            n127 = property class="GainBoost"(reference=w302, error in=w301, "Enabled"="Gain Boost") -> (reference out=w297:refnum<k24>, error out=w288:errorcluster)
            n128 = case "Snapshot control" shown="True" "Snapshot" {
              tunnel: w285 -> [_ w343]
              tunnel: w288 -> [w325 w347]
              tunnel: [w325 w334] -> w282
              tunnel: w284 -> [_ w337]
              tunnel: w283 -> [_ w336]
              frame False {
              }
              frame True {
                n129 = property class="Camera"(reference=w343, error in=w347) -> (error out=w367:errorcluster, "Memory"=w366:refnum<k24>)  [unwired: 1 out]
                n130 = local read "Zoom"() -> (w342:dbl)
                n131 = invoke class="Memory" method="GetList"(reference=w366, error in=w367) -> (reference out=w372:refnum<k24>, error out=w371:errorcluster, "GetList"=w373:i32, "idList"=w360:i32[])  [unwired: 2 in]
                n132 = Bundle(cluster=T2 {"Width"=0, "Height"=0} ("Draw Area Size"), "Width"=w337, "Height"=w336) -> (w338:T2)
                n133 = Divide(x=1.0, y=w342) -> (x/y=w340:dbl)
                n134 = property on="Output" class="Pict"("ZoomFactor"=w340, "Draw Area Size"=w338) -> ()  [unwired: 2 in, 2 out]
                n135 = invoke class="Memory" method="ToString"(reference=w372, error in=w371) -> (reference out=w345:refnum<k24>, error out=w355:errorcluster, "ToString"=w370:string)  [unwired: 1 in]
                n136 = Index Array(array=w360, index=0 ("Active \nAcquisition Buffer")) -> (element=w357:i32)
                n137 = Index Array(array=w360, index=u32 0 ("Active \nOutput Buffer")) -> (element=w356:i32)
                n138 = Close Reference(reference=w345, error in (no error)=w355) -> (error out=w354:errorcluster)
                n139 = Get Date/Time In Seconds() -> (seconds since 1Jan1904=w327:timestamp)
                n140 = call "uc480_Error_Handling.vi"("Error Code"=w373, "Error String"=w370, "Error In"=w354) -> ("Error Out"=w363:errorcluster)  [unwired: 8 in]
                n141 = property class="Camera"(reference=w343, error in=w363) -> (error out=w362:errorcluster, "Memory"=w361:refnum<k24>)  [unwired: 1 out]
                n142 = Format Date/Time String(time format string (%c)="%m/%d/%y -%I:%M %p  ", seconds (now)=w327) -> (date/time string=w326:string)  [unwired: 1 in]
                n143 = invoke class="Memory" method="SetActive"(reference=w361, error in=w362, "s32MemId"=w357) -> (reference out=w346:refnum<k24>, error out=w353:errorcluster)  [unwired: 1 in, 2 out]
                n144 = Concatenate Strings(w326, "Snapshot taken", "\r") -> (w331:string)
                n145 = Close Reference(reference=w346, error in (no error)=w353) -> (error out=w352:errorcluster)
                n146 = invoke on="Log" class="Str" method="Append String"("string"=w331) -> ()  [unwired: 3 in, 4 out]
                n147 = property class="Camera"(reference=w343, error in=w352) -> (error out=w369:errorcluster, "Memory"=w358:refnum<k24>)  [unwired: 1 out]
                n148 = invoke class="Memory" method="CopyToArray"(reference=w358, error in=w369, "s32MemId"=w356) -> (reference out=w348:refnum<k24>, error out=w349:errorcluster, "u8Image"=w368:u8[])  [unwired: 2 in, 2 out]
                n149 = invoke class="Memory" method="ToString"(reference=w348, error in=w349) -> (reference out=w344:refnum<k24>, error out=w351:errorcluster, "ToString"=w374:string)  [unwired: 1 in]
                n150 = Close Reference(reference=w344, error in (no error)=w351) -> (error out=w350:errorcluster)
                n151 = call "uc480_Error_Handling.vi"("Error String"=w374, "Error In"=w350) -> ("Error Out"=w365:errorcluster)  [unwired: 9 in]
                n152 = call "uc480_ArrayToImage.vi"("Error In"=w365, "InArray"=w368, ".NET (Reference)"=w343) -> ("Error Out"=w333:errorcluster, "Image"=w335:picture)  [unwired: 7 in]
                "Output" <- w335
                n153 = call "Picture to IMAQ.vi"("Error In"=w333, "picture"=w335) -> ("Error Out"=w334:errorcluster, "Image"=→"Source":T1)  [unwired: 8 in]
              }
            }
            n154 = Close Reference(reference=w296, error in (no error)=w282) -> (error out=w295:errorcluster)
            n155 = Close Reference(reference=w297, error in (no error)=w295) -> (error out=w292:errorcluster)
            n156 = Close Reference(reference=w304, error in (no error)=w292) -> (error out=w306:errorcluster)
            n157 = Close Reference(reference=w308, error in (no error)=w306) -> (error out=w320:errorcluster)
            n158 = Close Reference(reference=w318, error in (no error)=w320) -> (error out=w293:errorcluster)
          }
        }
      }
      frame "Init camera" {
        # "SubVI Example for \nGetDefault Timing"
        # "SubVI Example for \nMemory allocation"
        # "SubVI Example for \nTiming"
        # "SubVI Example for \nCamera Init"
        # "Pixelformat"
        n159 = control-ref of="Init Camera"() -> (w400:refnum<vi>)
        n160 = control-ref of="Load Parameter"() -> (w396:refnum<vi>)
        n161 = control-ref of="Start Live"() -> (w398:refnum<vi>)
        n162 = call "uc480_SubVI_Example_CameraInit.vi"("Error In"=w436, "Camera ID"="Camera ID", "Init Camera Flag"=TRUE, ".NET (Reference)"=w437) -> ("Error Out"=w442:errorcluster, ".NET (Reference)"=w395:refnum<k24>)  [unwired: 6 in]
        n163 = property class="Bool"(reference=w396, "Disabled"=u8 0 ("Deaktiviert")) -> (reference out=w385:refnum<vi>, error out=w384:errorcluster)  [unwired: 1 in]
        n164 = property class="Bool"(reference=w400, "Disabled"=u8 2 ("Deaktiviert")) -> (reference out=w389:refnum<vi>, error out=w388:errorcluster)  [unwired: 1 in]
        n165 = property class="Bool"(reference=w398, "Disabled"=u8 0 ("Deaktiviert")) -> (reference out=w387:refnum<vi>, error out=w386:errorcluster)  [unwired: 1 in]
        n166 = property on="Property Node" class="Camera"(reference=w395, error in=w442) -> (error out=w443:errorcluster, "PixelFormat"=w444:refnum<k24>)  [unwired: 1 out]
        n167 = Close Reference(reference=w389, error in (no error)=w388) -> ()  [unwired: 1 out]
        n168 = Close Reference(reference=w387, error in (no error)=w386) -> ()  [unwired: 1 out]
        n169 = Close Reference(reference=w385, error in (no error)=w384) -> ()  [unwired: 1 out]
        n170 = invoke class="PixelFormat" method="Set"(reference=w444, error in=w443, "mode"="Mode") -> (reference out=w440:refnum<k24>, error out=w433:errorcluster, "Set"=w439:i32)  [unwired: 1 in, 1 out]
        n171 = invoke class="PixelFormat" method="ToString"(reference=w440, error in=w433) -> (reference out=w381:refnum<k24>, error out=w383:errorcluster, "ToString"=w441:string)  [unwired: 1 in]
        n172 = Close Reference(reference=w381, error in (no error)=w383) -> (error out=w382:errorcluster)
        n173 = call "uc480_Error_Handling.vi"("Error Code"=w439, "Error String"=w441, "Error In"=w382) -> ("Error Out"=w407:errorcluster)  [unwired: 8 in]
        n174 = call "uc480_SubVI_Example_GetDefault_Timing.vi"(".NET (Reference)"=w395, "Error In"=w407) -> ("Pixelclock"=w406:i32, "Exposure time"=w405:dbl, "Framerate"=w404:dbl, "Error Out"=w403:errorcluster)  [unwired: 10 in]
        n175 = call "uc480_SubVI_Example_GetPixelClock.vi"(".NET (Reference)"=w395, "Error In"=w403) -> ("Pixel Clock"=w408:i32, "Inc"=w410:i32, "Min"=w411:i32, "Max"=w412:i32, "error out"=w409:errorcluster)  [unwired: 9 in]
        n176 = property on="Pixelclock" class="Slide (strict)"(error in=w409, "Value"=w408, "Increment"=w410, "Minimum"=w411, "Maximum"=w412) -> (error out=w413:errorcluster)  [unwired: 1 in, 1 out]
        n177 = property on="Pixelclock" class="Slide (strict)"(error in=w413, "Scale.Increment"=w410, "Scale.Minimum"=w411, "Scale.Maximum"=w412) -> (error out=w414:errorcluster)  [unwired: 1 in, 1 out]
        n178 = call "uc480_SubVI_Example_GetFramerate.vi"(".NET (Reference)"=w395, "Error In"=w414) -> ("Framerate"=w417:dbl, "Inc"=w418:dbl, "Min"=w419:dbl, "Max"=w420:dbl, "error out"=w416:errorcluster)  [unwired: 9 in]
        n179 = property on="Framerate" class="Slide (strict)"(error in=w416, "Value"=w417, "Increment"=w418, "Minimum"=w419, "Maximum"=w420) -> (error out=w415:errorcluster)  [unwired: 1 in, 1 out]
        n180 = property on="Framerate" class="Slide (strict)"(error in=w415, "Scale.Increment"=w418, "Scale.Minimum"=w419, "Scale.Maximum"=w420) -> (error out=w421:errorcluster)  [unwired: 1 in, 1 out]
        n181 = call "uc480_SubVI_Example_GetExposure.vi"(".NET (Reference)"=w395, "Error In"=w421) -> ("Exposure"=w424:dbl, "Inc"=w425:dbl, "Min"=w426:dbl, "Max"=w427:dbl, "Error out"=w422:errorcluster)  [unwired: 9 in]
        n182 = property on="Exposure" class="Slide (strict)"(error in=w422, "Value"=w424, "Increment"=w425, "Minimum"=w426, "Maximum"=w427) -> (error out=w423:errorcluster)  [unwired: 1 in, 1 out]
        n183 = property on="Exposure" class="Slide (strict)"(error in=w423, "Scale.Increment"=w425, "Scale.Minimum"=w426, "Scale.Maximum"=w427) -> (error out=w402:errorcluster)  [unwired: 1 in, 1 out]
        n184 = call "uc480_SubVI_Example_Timing.vi"(".NET (Reference)"=w395, "Pixelclock"=w406, "Exposure time"=w405, "Framerate"=w404, "Error In"=w402) -> ("Error Out"=w394:errorcluster)  [unwired: 7 in, 3 out]
        n185 = call "uc480_SubVI_Example_Is_XS.vi"("Error In"=w394, ".NET (Reference)"=w395) -> ("Error Out"=w391:errorcluster, "IsXS"=w393:bool)  [unwired: 7 in, 1 out]
        n186 = case shown="False" w393 {
          tunnel: w391 -> [w458 w471]
          tunnel: [w458 w471] -> w392
          frame False {
            n187 = control-ref of="Pixelclock"() -> (w454:refnum<vi>)
            n188 = control-ref of="Framerate"() -> (w453:refnum<vi>)
            n189 = control-ref of="Exposure"() -> (w452:refnum<vi>)
            n190 = property class="Slide (strict)"(reference=w454, "DisabledEnum"=T3."Enabled" ("Disabled")) -> (reference out=w451:refnum<vi>, error out=w450:errorcluster)  [unwired: 1 in]
            n191 = property class="Slide (strict)"(reference=w453, "DisabledEnum"=T3."Enabled" ("Disabled")) -> (reference out=w449:refnum<vi>, error out=w448:errorcluster)  [unwired: 1 in]
            n192 = property class="Slide (strict)"(reference=w452, "DisabledEnum"=T3."Enabled" ("Disabled")) -> (reference out=w447:refnum<vi>, error out=w446:errorcluster)  [unwired: 1 in]
            n193 = Close Reference(reference=w447, error in (no error)=w446) -> ()  [unwired: 1 out]
            n194 = Close Reference(reference=w451, error in (no error)=w450) -> ()  [unwired: 1 out]
            n195 = Close Reference(reference=w449, error in (no error)=w448) -> ()  [unwired: 1 out]
          }
          frame True {
            n196 = control-ref of="Pixelclock"() -> (w470:refnum<vi>)
            n197 = control-ref of="Framerate"() -> (w467:refnum<vi>)
            n198 = control-ref of="Exposure"() -> (w465:refnum<vi>)
            n199 = property class="Slide (strict)"(reference=w470, "DisabledEnum"=T3."Disabled and Grayed Out" ("Disabled")) -> (reference out=w463:refnum<vi>, error out=w464:errorcluster)  [unwired: 1 in]
            n200 = property class="Slide (strict)"(reference=w467, "DisabledEnum"=T3."Disabled and Grayed Out" ("Disabled")) -> (reference out=w462:refnum<vi>, error out=w461:errorcluster)  [unwired: 1 in]
            n201 = property class="Slide (strict)"(reference=w465, "DisabledEnum"=T3."Disabled and Grayed Out" ("Disabled")) -> (reference out=w460:refnum<vi>, error out=w459:errorcluster)  [unwired: 1 in]
            n202 = Close Reference(reference=w462, error in (no error)=w461) -> ()  [unwired: 1 out]
            n203 = Close Reference(reference=w460, error in (no error)=w459) -> ()  [unwired: 1 out]
            n204 = Close Reference(reference=w463, error in (no error)=w464) -> ()  [unwired: 1 out]
          }
        }
        n205 = call "uc480_SubVI_Example_MemoryAllocation.vi"(".NET (Reference)"=w395, "Error In"=w392) -> ("Bits/Pixel 2"=→"Bits/Pixel":i32, "Width"=→"Width":i32, "Serial Number"=→"Serial Number":string, "Height"=→"Height":i32, "Error Out"=w432:errorcluster)  [unwired: 13 in]
        n206 = Get Date/Time In Seconds() -> (seconds since 1Jan1904=w376:timestamp)
        n207 = Format Date/Time String(time format string (%c)="%m/%d/%y -%I:%M %p  ", seconds (now)=w376) -> (date/time string=w375:string)  [unwired: 1 in]
        n208 = Concatenate Strings(w375, "Camera Initialized", "\r") -> (w380:string)
        n209 = invoke on="Log" class="Str" method="Append String"("string"=w380) -> ()  [unwired: 3 in, 4 out]
      }
      frame "Start live" {
        # "Has acquisition started?"
        # "Start Acquisition"
        n210 = control-ref of="Start Live"() -> (w490:refnum<vi>)
        n211 = control-ref of="Load Parameter"() -> (w487:refnum<vi>)
        n212 = control-ref of="Stop Live"() -> (w485:refnum<vi>)
        n213 = property class="Bool (strict)"(reference=w485, "Disabled"=u8 0 ("Deaktiviert")) -> (reference out=w483:refnum<vi>, error out=w482:errorcluster)  [unwired: 1 in]
        n214 = property class="Bool"(reference=w490, "Disabled"=u8 2 ("Deaktiviert")) -> (reference out=w479:refnum<vi>, error out=w478:errorcluster)  [unwired: 1 in]
        n215 = property class="Bool"(reference=w487, "Disabled"=u8 2 ("Deaktiviert")) -> (reference out=w481:refnum<vi>, error out=w480:errorcluster)  [unwired: 1 in]
        n216 = Close Reference(reference=w481, error in (no error)=w480) -> ()  [unwired: 1 out]
        n217 = Close Reference(reference=w479, error in (no error)=w478) -> ()  [unwired: 1 out]
        n218 = Close Reference(reference=w483, error in (no error)=w482) -> ()  [unwired: 1 out]
        n219 = property class="Camera"(reference=w494, error in=w495) -> (error out=w504:errorcluster, "Acquisition"=w503:refnum<k24>)  [unwired: 1 out]
        n220 = invoke class="Acquisition" method="HasStarted"(reference=w503, error in=w504) -> (reference out=w499:refnum<k24>, error out=w498:errorcluster, "HasStarted"=w497:i32, "bValue"=w502:bool)  [unwired: 2 in]
        n221 = invoke class="Acquisition" method="ToString"(reference=w499, error in=w498) -> (error out=w501:errorcluster, "ToString"=w500:string)  [unwired: 1 in, 1 out]
        n222 = call "uc480_Error_Handling.vi"("Error Code"=w497, "Error String"=w500, "Error In"=w501) -> ("Error Out"=w496:errorcluster)  [unwired: 8 in]
        n223 = case shown="False" w502 {
          tunnel: [w507 w517] -> w491
          tunnel: w496 -> [w513 w517]
          tunnel: w494 -> [w512 w516]
          tunnel: [w512 w516] -> w493
          frame False {
            w505 = 1 items=["IS_DONT_WAIT", "IS_WAIT"] ("Wait")
            n224 = property class="Camera"(reference=w512, error in=w513) -> (error out=w514:errorcluster, "Acquisition"=w515:refnum<k24>)  [unwired: 1 out]
            n225 = invoke class="Acquisition" method="Capture"(reference=w515, error in=w514, "param"=w505) -> (reference out=w508:refnum<k24>, error out=w509:errorcluster, "Capture"=w506:i32)  [unwired: 1 in, 1 out]
            n226 = invoke class="Acquisition" method="ToString"(reference=w508, error in=w509) -> (error out=w511:errorcluster, "ToString"=w510:string)  [unwired: 1 in, 1 out]
            n227 = call "uc480_Error_Handling.vi"("Error Code"=w506, "Error String"=w510, "Error In"=w511) -> ("Error Out"=w507:errorcluster)  [unwired: 8 in]
          }
          frame True {
          }
        }
        n228 = Get Date/Time In Seconds() -> (seconds since 1Jan1904=w473:timestamp)
        n229 = Format Date/Time String(time format string (%c)="%m/%d/%y -%I:%M %p  ", seconds (now)=w473) -> (date/time string=w472:string)  [unwired: 1 in]
        n230 = Concatenate Strings(w472, "Camera started", "\r") -> (w477:string)
        n231 = invoke on="Log" class="Str" method="Append String"("string"=w477) -> ()  [unwired: 3 in, 4 out]
      }
    }
    n232 = call "uc480_SubVI_Example_SyncEventLoop.vi"("Error In"=w34, "use sync"=w36, ".NET (Reference)"=w35) -> ("Error Out"=w32:errorcluster, "Synchronize (ms)"=w33:dbl)  [unwired: 7 in]
    "Error Out" <- w32
    n233 = Wait Until Next ms Multiple(millisecond multiple=w33) -> ()  [unwired: 1 out]
  }
  n234 = property class="Bool"(reference=w25, "Disabled"=u8 0 ("Deaktiviert")) -> (reference out=w13:refnum<vi>, error out=w12:errorcluster)  [unwired: 1 in]
  n235 = property class="Bool"(reference=w22, "Disabled"=u8 2 ("Deaktiviert")) -> (reference out=w11:refnum<vi>, error out=w10:errorcluster)  [unwired: 1 in]
  n236 = Close Reference(reference=w11, error in (no error)=w10) -> ()  [unwired: 1 out]
  n237 = Close Reference(reference=w13, error in (no error)=w12) -> ()  [unwired: 1 out]
  n238 = control-ref of="Load Parameter"() -> (w19:refnum<vi>)
  n239 = control-ref of="Stop Live"() -> (w18:refnum<vi>)
  n240 = flat-sequence "Initialization sequence" {
    tunnel: [w555] -> w26
    tunnel: w26 -> [w598]
    frame #0 {
      # "Put name of .ini file here (i.e., opotek_27015_849_847.ini).\nThe .ini file must be in the 'c:\\opotek' directory"
      n241 = control-ref of="This VI"() -> (w542:refnum<vi>)
      n242 = invoke class="VI" method="Default Vals.Reinit All"(reference=w542) -> ()  [unwired: 2 in, 3 out]
      n243 = call "File Dialog"("start path"=path "C:/opotek", "pattern (all files)"="*.ini*") -> ("selected path"=w539:path, "cancelled"=w538:bool, "error out"=w537:errorcluster)  [unwired: 10 in, 1 out]
      n244 = case shown="False" w538 {
        tunnel: w537 -> [w551 w553]
        tunnel: [w551 w552] -> w536
        frame False {
          n245 = Get Date/Time In Seconds() -> (seconds since 1Jan1904=w546:timestamp)
          n246 = Format Date/Time String(time format string (%c)="%m/%d/%y -%I:%M %p  ", seconds (now)=w546) -> (date/time string=w545:string)  [unwired: 1 in]
          n247 = Concatenate Strings(w545, "Initializing the OPO laser..." ("Initialiazation"), "\r") -> (w550:string)
          n248 = invoke on="Log" class="Str" method="Append String"("string"=w550) -> ()  [unwired: 3 in, 4 out]
        }
        frame True {
          n249 = call <vilib>:"Clear Errors.vi"("error in (no error)"=w553) -> ("error out"=w552:errorcluster)  [unwired: 5 in, 1 out]
        }
      }
      n250 = Strip Path(path=w539) -> (name=w543:string)  [unwired: 1 out]
      n251 = dll-call lib="D:/Fabrizio/Labview Projects/IR OPO Controller/Branches/Final version/OPOTEK.dll" fn="OPOTEK_Init"("INI_File"=w543) -> ("motorCOMPort"=w535:i32, "laserCOMPort"=w534:i32, "error_Code"=→"error_Code":i32)  [unwired: 8 in, 2 out]
      "motorCOMPort" <- w535
      "laserCOMPort" <- w534
      n252 = Number To Decimal String(number=w535) -> (decimal integer string=w533:string)  [unwired: 1 in]
      n253 = Number To Decimal String(number=w534) -> (decimal integer string=w531:string)  [unwired: 1 in]
      n254 = Concatenate Strings("Motor found on port: " ("string"), w533) -> (w529:string)
      n255 = Concatenate Strings("Laser found on port: " ("string"), w531) -> (w528:string)
      n256 = Build Array(w529) -> (w527:string[])
      n257 = Build Array(w528) -> (w526:string[])
      n258 = Build Array(w527, w526) -> (w525:string[][])
      n259 = Array To Spreadsheet String(array=w525, 3:"%s" ("format string")) -> (spreadsheet string=w522:string)  [unwired: 1 in]
      n260 = Get Date/Time In Seconds() -> (seconds since 1Jan1904=w519:timestamp)
      n261 = Format Date/Time String(time format string (%c)="%m/%d/%y -%I:%M %p  ", seconds (now)=w519) -> (date/time string=w518:string)  [unwired: 1 in]
      n262 = Concatenate Strings(w518, w522, "\r") -> (w523:string)
      n263 = call <vilib>:"Simple Error Handler.vi"("error in (no error)"=w536) -> ()  [unwired: 4 in, 5 out]
      n264 = invoke on="Log" class="Str" method="Append String"("string"=w523) -> ()  [unwired: 3 in, 4 out]
    }
    frame #1 {
      w554 = "Communication" ("section")
      n265 = control-ref of="This VI"() -> (w586:refnum<vi>)
      n266 = property class="VI"(reference=w586) -> ("Path"=w583:path)  [unwired: 1 in, 2 out]
      n267 = Strip Path(path=w583) -> (stripped path=w582:path)  [unwired: 1 out]
      n268 = Build Path(base path=w582, name or relative path="ESP_GPIB_Config.ini") -> (appended path=w570:path)
      n269 = call <vilib>:"Open Config Data.vi"("create file if necessary (T)"=FALSE, "configuration file path"=w570) -> ("error out"=w587:errorcluster, "refnum"=w584:T4)  [unwired: 7 in, 1 out]
      n270 = call <vilib>:"Open Config Data.vi"("create file if necessary (T)"=FALSE, "configuration file path"=w570) -> ("error out"=w578:errorcluster, "refnum"=w577:T4)  [unwired: 7 in, 1 out]
      n271 = call <vilib>:"Open Config Data.vi"("create file if necessary (T)"=FALSE, "configuration file path"=w570) -> ("error out"=w575:errorcluster, "refnum"=w574:T4)  [unwired: 7 in, 1 out]
      n272 = call <vilib>:"Open Config Data.vi"("create file if necessary (T)"=FALSE, "configuration file path"=w570) -> ("error out"=w572:errorcluster, "refnum"=w571:T4)  [unwired: 7 in, 1 out]
      n273 = call-poly <vilib>:"Read Key.vi"("section"=w554, "error in (no error)"=w587, "default value"=0, "key"="GPIBport", "refnum"=w584) -> ("error out"=w556:errorcluster, "value"=→"GPIBport":i32)  [unwired: 3 in, 2 out]
      n274 = call-poly <vilib>:"Read Key.vi"("section"=w554, "error in (no error)"=w578, "default value"=0, "key"="GPIBdelay", "refnum"=w577) -> ("error out"=w557:errorcluster, "value"=→"GPIBdelay":i32)  [unwired: 3 in, 2 out]
      n275 = call-poly <vilib>:"Read Key.vi"("section"=w554, "error in (no error)"=w575, "default value"=300, "key"="GPIBtimeout", "refnum"=w574) -> ("error out"=w558:errorcluster, "value"=→"GPIBtimeout":i32)  [unwired: 3 in, 2 out]
      n276 = call-poly <vilib>:"Read Key.vi"("section"=w554, "error in (no error)"=w572, "default value"=0, "key"="GPIBtermchar", "refnum"=w571) -> ("error out"=w559:errorcluster, "value"=→"GPIBtermChar":i32)  [unwired: 3 in, 2 out]
      n277 = Merge Errors(w556, w557, w558, w559) -> (w555:errorcluster)
    }
    frame #2 {
      n278 = local read "GPIB Mode"() -> (w595:i16)
      n279 = local read "GPIBport"() -> (w599:i32)
      n280 = call "esp_gpib_send_ASCII.vi"("mode (0)"=w595, "ASCII Cmd"="tb?", "error in"=w598, "Port In"=w599) -> ("Status Out"=w596:i32, "Port Out"=w597:i32)  [unwired: 3 in, 3 out]
      n281 = call "esp_gpib_read_ASCII.vi"("Port In"=w597, "Status In"=w596) -> ("StringOut"=w592:string, "error out"=w601:errorcluster)  [unwired: 3 in, 3 out]
      n282 = call <vilib>:"Simple Error Handler.vi"("error in (no error)"=w601) -> ("error?"=w602:bool)  [unwired: 4 in, 4 out]
      n283 = Get Date/Time In Seconds() -> (seconds since 1Jan1904=w590:timestamp)
      n284 = Stop(stop? (T)=w602) -> ()
      n285 = Format Date/Time String(time format string (%c)="%m/%d/%y -%I:%M %p  ", seconds (now)=w590) -> (date/time string=w589:string)  [unwired: 1 in]
      n286 = Concatenate Strings(w589, w592, "\r") -> (w594:string)
      n287 = invoke on="Log" class="Str" method="Append String"("string"=w594) -> ()  [unwired: 3 in, 4 out]
    }
    frame #3 {
      n288 = dll-call lib="D:/Fabrizio/Labview Projects/IR OPO Controller/Branches/Final version/OPOTEK.dll" fn="OPOTEK_SelectConfiguration"("configuration"=u8 1 ("configuration 2")) -> ("wavelength_Low"=→"Min":dbl, "wavelength_High"=→"Max":dbl, "error_Code"=→"error_Code 2":i32)  [unwired: 8 in, 2 out]
    }
    frame #4 {
      w609 = FALSE ("Visible")
      w614 = u8 1 ("Response to Value Outside Limits:Maximum")
      # "Set defaults"
      n289 = local write "Repetition \nRate"(enum16{"1", "2", "5", "10", "20"}."20" ("Rep. Rate Divider")) -> ()
      n290 = local read "Max"() -> (w617:dbl)
      n291 = local read "Min"() -> (w616:dbl)
      n292 = property on="LASER" class="Bool (strict)"("BoolText.Text"="LASER OFF" ("Boolean Text.Text"), "Visible"=FALSE) -> ()  [unwired: 2 in, 2 out]
      n293 = property on="Wavelength" class="DigNum (strict)"("Increment"=1.0 ("Data Entry Limits:Increment"), "Maximum"=w617, "Minimum"=w616, "OutOfRngActMax"=w614, "OutOfRngActMin"=w614) -> ()  [unwired: 2 in, 2 out]
      n294 = call "IR_Alignment_Diode.vi"("AD Action"=enum16{"AD Off", "AD On"}."AD On") -> ()  [unwired: 14 in, 1 out]
      n295 = property on="LAMP" class="Bool (strict)"("BoolText.Text"="LAMP OFF" ("Boolean Text.Text")) -> ()  [unwired: 2 in, 2 out]
      n296 = property on="Capture" class="Bool"("Visible"=w609) -> ()  [unwired: 2 in, 2 out]
      n297 = property on="Laser Operation" class="Bool (strict)"("Blinking"=w609) -> ()  [unwired: 2 in, 2 out]
      n298 = Add(x=w617, y=w616) -> (x+y=w621:dbl)
      n299 = local write "Alignment \ndiode"(TRUE ("Alignment diode")) -> ()
      n300 = local write "Energy (%)"(i16 0 ("Energy")) -> ()
      n301 = Divide(x=w621, y=2.0) -> (x/y=w611:dbl)
      n302 = local write "Wavelength"(w611) -> ()
      n303 = property on="Current Wavelength" class="DigNum (strict)"("Value"=w611) -> ()  [unwired: 2 in, 2 out]
      n304 = call "IR_Wavelength_Tuning.vi"("Wavelength (nm)"=w611) -> ()  [unwired: 14 in, 1 out]
    }
  }
  n305 = property class="Bool (strict)"(reference=w18, "Disabled"=u8 2 ("Deaktiviert")) -> (reference out=w9:refnum<vi>, error out=w8:errorcluster)  [unwired: 1 in]
  n306 = property class="Bool"(reference=w19, "Disabled"=u8 2 ("Deaktiviert")) -> (reference out=w7:refnum<vi>, error out=w6:errorcluster)  [unwired: 1 in]
  n307 = Close Reference(reference=w7, error in (no error)=w6) -> ()  [unwired: 1 out]
  n308 = Close Reference(reference=w9, error in (no error)=w8) -> ()  [unwired: 1 out]
  n309 = while "ROI Processing" {
    stop <- w628 stop-if-true
    n310 = event shown="[1] \"Process Image\": Value Change" {
      selector: _ -> [_ _]
      dyn-events: _ -> [_ _]
      timeout: _ -> [_ _]
      tunnel: ["EXIT 3" _] -> w628
      tunnel: [_ w679] -> w625
      event "EXIT": Value Change {
        n311 = event-data() -> ()  [unwired: 1 in, 6 out]
      }
      event "Process Image": Value Change {
        w656 = T5 0 items=["Grayscale (U8)", "Grayscale (I16)", "Grayscale (SGL)", "Complex (CSG)", "RGB (U32)", "HSL (U32)", "RGB (U64)", "Grayscale (U16)"] ("Image Type")
        w661 = i16 3 ("precision (6)")
        w642 = 1000 ("y")
        # "to change to X*Y"
        # "This double loop parses the ROI with a subarray equal to the size of the laser spot diameter."
        n312 = event-data() -> ()  [unwired: 1 in, 6 out]
        n313 = local read "Source"() -> (w658:T1)
        n314 = property on="Source" class="ImageControl"() -> ("ROI"=w668:T6)  [unwired: 2 in, 2 out]
        n315 = local read "Laser spot\nY diameter"() -> (w640:i32)
        n316 = local read "Laser spot\nX diameter"() -> (w637:i32)
        n317 = local read "Pixel \nsize"() -> (w662:dbl)
        n318 = Unbundle By Name(w668) -> ("Global Rectangle"=w667:i32[])
        n319 = call "IMAQ Cast Image"("Image Type"=w656, "Image Src"=w658) -> ("Image Dst Out"=w657:T1)  [unwired: 8 in, 1 out]
        n320 = local read "Laser offset \nY Position"() -> (w654:i32)
        n321 = local read "Laser offset \nX Position"() -> (w652:i32)
        n322 = local read "Y axis \nprecision"() -> (w681:i32)
        n323 = Add(x=w640, y=w637) -> (x+y=w641:i32)
        n324 = call "IMAQ ROIToMask 2"("ROI Descriptor"=w668, "Image"=w657) -> ("Image Out"=w672:T1)  [unwired: 7 in, 2 out]
        n325 = Index Array(array=w667, index=1) -> (element=w655:i32)
        "ROI Rectangle Y position" <- w655
        n326 = Index Array(array=w667, index=0) -> (element=w653:i32)
        "ROI Rectangle X position" <- w653
        n327 = Subtract(x=w655, y=w654) -> (x-y=w663:i32)
        n328 = Subtract(x=w653, y=w652) -> (x-y=w664:i32)
        n329 = call "IMAQ ImageToArray"("Image"=w672) -> ("Image Pixels (U8)"=w671:u8[][])  [unwired: 3 in, 4 out]
        n330 = Quotient & Remainder(x=w641, y=2) -> (floor(x/y)=w638:i32)  [unwired: 1 out]
        n331 = local read "Axes speed \n(µm/s)"() -> (w670:i32)
        n332 = Multiply(x=w663, y=w662) -> (x*y=w644:dbl)
        n333 = Multiply(x=w664, y=w662) -> (x*y=w643:dbl)
        n334 = Quotient & Remainder(x=w638, y=w662) -> (floor(x/y)=w684:dbl)  [unwired: 1 out]
        n335 = Array Size(array=w671) -> (size(s)=w714:i32[])
        n336 = Array Size(array=w671) -> (size(s)=w673:i32[])
        n337 = Divide(x=w684, y=w681) -> (x/y=w636:dbl)
        n338 = Divide(x=w640, y=w681) -> (x/y=w682:dbl)
        n339 = Square(x=w684) -> (x^2=→"# pixels in an ablation spot":dbl)
        n340 = Array To Cluster(array=w673) -> (cluster=w674:cluster{"[0]":i32, "[1]":i32})
        n341 = Less?(x=w644, y=0.0) -> (x < y?=w646:bool)
        n342 = Less?(x=w643, y=0.0) -> (x < y?=w650:bool)
        n343 = Index Array(array=w714, index=0) -> (element=w712:i32)
        n344 = Index Array(array=w714, index=1) -> (element=w716:i32)
        n345 = Subtract(x=w716, y=w684) -> (x-y=w715:dbl)
        n346 = Subtract(x=w712, y=w684) -> (x-y=w711:dbl)
        n347 = Divide(x=w682, y=w670) -> (x/y=w688:dbl)
        n348 = Round To Nearest(number=w636) -> (nearest integer value=w683:dbl)
        n349 = Unbundle(w674) -> ("[0]"=w678:i32, "[1]"=w677:i32)
        "Y size \n(pixels)" <- w678
        "X size\n(pixels)" <- w677
        n350 = case shown="False" w646 {
          tunnel: w644 -> [w722 w730]
          tunnel: [w719 w726] -> w647
          tunnel: w640 -> [w724 w729]
          tunnel: w642 -> [w720 w728]
          frame False {
            n351 = Divide(x=w724, y=2) -> (x/y=w723:dbl)
            n352 = Add(x=w722, y=w723) -> (x+y=w721:dbl)
            n353 = Divide(x=w721, y=w720) -> (x/y=w719:dbl)
          }
          frame True {
            n354 = Divide(x=w729, y=2) -> (x/y=w731:dbl)
            n355 = Subtract(x=w730, y=w731) -> (x-y=w727:dbl)
            n356 = Divide(x=w727, y=w728) -> (x/y=w726:dbl)
          }
        }
        n357 = case shown="True" w650 {
          tunnel: w643 -> [w736 w744]
          tunnel: [w733 w740] -> w648
          tunnel: w637 -> [w738 w743]
          tunnel: w642 -> [w735 w742]
          frame False {
            n358 = Divide(x=w738, y=2) -> (x/y=w737:dbl)
            n359 = Add(x=w736, y=w737) -> (x+y=w734:dbl)
            n360 = Divide(x=w734, y=w735) -> (x/y=w733:dbl)
          }
          frame True {
            n361 = Divide(x=w743, y=2) -> (x/y=w745:dbl)
            n362 = Subtract(x=w744, y=w745) -> (x-y=w741:dbl)
            n363 = Divide(x=w741, y=w742) -> (x/y=w740:dbl)
          }
        }
        n364 = local read "Fast \nsampling?"() -> (w680:bool)
        n365 = To Long Integer(number=w683) -> (32bit integer=w635:i32)
        "Y step size in pixels" <- w635
        n366 = Multiply(x=w688, y=1000.0) -> (x*y=w686:dbl)
        n367 = Multiply(x=w662, y=w635) -> (x*y=→"Y Step size in µm":dbl)
        n368 = Multiply(x=w678, y=w662) -> (x*y=→"Y size \n(µm)":dbl)
        n369 = Multiply(x=w677, y=w662) -> (x*y=→"X size \n(µm)":dbl)
        n370 = case shown="True" w680 {
          tunnel: w711 -> [w851 w856]
          tunnel: [w851 w853] -> w710
          tunnel: w635 -> [_ w852]
          frame False {
          }
          frame True {
            n371 = Quotient & Remainder(x=w856, y=w852) -> (floor(x/y)=w855:dbl)  [unwired: 1 out]
            n372 = Add(x=w855, y=1) -> (x+y=w853:dbl)
          }
        }
        n373 = Round To Nearest(number=w686) -> (nearest integer value=→"Y axis moving time":dbl)
        n374 = Number To Fractional String(number=w647, precision (6)=w661) -> (F-format string=→"Laser Y offset":string)  [unwired: 2 in]
        n375 = Number To Fractional String(number=w648, precision (6)=w661) -> (F-format string=→"Laser X offset":string)  [unwired: 2 in]
        n376 = for {
          N: w710 -> [_]
          tunnel: w671 -> [w864]
          tunnel: w715 -> [w863]
          tunnel: w684 -> [w862]
          tunnel: [w861] -> w708 mode=indexing
          tunnel: w680 -> [w858]
          tunnel: w635 -> [w857]
          i -> [w860]
          n377 = case shown="True" w858 {
            tunnel: w860 -> [w865 w868]
            tunnel: [w865 w867] -> w859
            tunnel: w857 -> [_ w866]
            frame False {
            }
            frame True {
              n378 = Multiply(x=w868, y=w866) -> (x*y=w867:i32)
            }
          }
          n379 = for {
            N: w863 -> [_]
            tunnel: w862 -> [w874]
            tunnel: w859 -> [w876]
            tunnel: w864 -> [w875]
            tunnel: [w872] -> w861 mode=indexing
            i -> [w870]
            n380 = for {
              N: w874 -> [_]
              tunnel: w875 -> [w888]
              tunnel: [w887] -> w869 mode=indexing
              tunnel: w874 -> [w886]
              tunnel: w876 -> [w885]
              tunnel: w870 -> [w882]
              i -> [w884]
              n381 = Add(x=w885, y=w884) -> (x+y=w883:i32)
              n382 = for {
                N: w886 -> [_]
                tunnel: w888 -> [w894]
                tunnel: [w893] -> w887 mode=indexing
                tunnel: w883 -> [w892]
                tunnel: w882 -> [w890]
                i -> [w891]
                n383 = Add(x=w890, y=w891) -> (x+y=w889:i32)
                n384 = Index Array(array=w894, index (row)=w892, index (col)=w889) -> (element=w893:u8)
              }
            }
            n385 = local read "# pixels in an ablation spot"() -> (w873:i32)
            n386 = Equal?(x=w869, y=255.0) -> (x = y?=w880:bool[][])
            n387 = Boolean To (0,1)(Boolean=w880) -> (0, 1=w879:i16[][])
            n388 = Add Array Elements(numeric array=w879) -> (sum=w878:i16)
            n389 = Divide(x=w878, y=w873) -> (x/y=w871:dbl)
            n390 = Greater Or Equal?(x=w871, y="Sampling\nPrecision") -> (x >= y?=w872:bool)
          }
        }
        n391 = Index Array(array=w708, index (col)=0 ("disabled index (col)")) -> (element=w706:bool[])  [unwired: 1 in]
        n392 = Array Size(array=w706) -> (size(s)=w707:i32)
        n393 = for {
          N: w707 -> [_]
          tunnel: w708 -> [w817]
          tunnel: [w815] -> w705 mode=indexing
          tunnel: [w814] -> w630 mode=indexing
          i -> [w820]
          # "This loop transform the 2D boolean array in a 1D boolean array alternating the lines in order to replicate the serpentine pattern of the axes\nIt also adds the pixels for the Y axis movement"
          n394 = Index Array(array=w817, index (row)=w820) -> (element=w818:bool[])  [unwired: 1 in]
          n395 = Quotient & Remainder(x=w820, y=2) -> (x-y*floor(x/y)=w822:i32)  [unwired: 1 out]
          n396 = Equal To 0?(x=w822) -> (x = 0?=w819:bool)
          n397 = case shown="False" w819 {
            tunnel: w818 -> [w849 w850]
            tunnel: [w848 w850] -> w816
            frame False {
              n398 = Reverse 1D Array(array=w849) -> (reversed array=w848:bool[])
            }
            frame True {
            }
          }
          n399 = while {
            tunnel: w816 -> [w837]
            tunnel: [w842] -> w815 mode=indexing
            tunnel: [w823] -> w814 mode=indexing
            i -> [w834]
            stop <- w826 stop-if-true
            # "This while loop counts the  number of consecutive T or F values and sort them in an array. Each number needs to be multiplied by the delta time in order to have a timed array that is aligned with the axes array"
            n400 = Greater?(x=w834, y=0) -> (0:w835:bool)
            n401 = feedback #1() -> (w836:bool[])  [unwired: 1 in]
            n402 = case shown="True" w835 {
              tunnel: w837 -> [w846 _]
              tunnel: [w846 w847] -> w827
              tunnel: w836 -> [_ w847]
              frame False {
              }
              frame True {
              }
            }
            n403 = And Array Elements(Boolean array=w827) -> (logical AND=w831:bool)
            n404 = Or Array Elements(Boolean array=w827) -> (logical OR=w829:bool)
            n405 = Index Array(array=w827, index=0) -> (element=w840:bool)
            n406 = Not(x=w829) -> (.not. x?=w828:bool)
            n407 = Not(x=w840) -> (.not. x?=w839:bool)
            n408 = Or(x=w831, y=w828) -> (x .or. y?=w826:bool)
            n409 = Search 1D Array(1D array=w827, element=w839, start index (0)=0) -> (index of element=w838:i32)
            n410 = Split 1D Array(array=w827, index=w838) -> (first subarray=w830:bool[], second subarray=w832:bool[])
            n411 = feedback-in #1(w832) -> ()
            n412 = case shown="True" w826 {
              tunnel: w830 -> [w844 _]
              tunnel: [w844 w845] -> w825
              tunnel: w827 -> [_ w845]
              frame False {
              }
              frame True {
              }
            }
            n413 = Array Size(array=w825) -> (size(s)=w842:i32)
            n414 = Index Array(array=w825, index=0) -> (element=w823:bool)
          }
        }
        n415 = for {
          tunnel: w705 -> [w812] mode=indexing
          tunnel: [w811] -> w669 mode=indexing
          n416 = local read "Pixel \nsize"() -> (w813:dbl)
          n417 = Multiply(x=w813, y=w812) -> (x*y=w811:dbl[])
        }
        n418 = Index Array(array=w630, index (col)=0 ("disabled index (col)")) -> (element=w696:bool[])  [unwired: 1 in]
        n419 = Array Size(array=w696) -> (size(s)=w695:i32)
        n420 = for {
          N: w695 -> [_]
          tunnel: w630 -> [w757] mode=indexing
          tunnel: [w755] -> w694 mode=indexing
          # "This loop add a F for each Y moviment"
          n421 = Build Array (concatenate)(w757, FALSE) -> (w755:bool[])
        }
        "Laser on/off array" <- w694
        n422 = Index Array(array=w669, index (col)=0 ("disabled index (col)")) -> (element=w701:dbl[])  [unwired: 1 in]
        n423 = Index Array(array=w669, index (row)=0) -> (element=w703:dbl[])  [unwired: 1 in]
        n424 = Array Size(array=w701) -> (size(s)=w699:i32)
        n425 = Array Size(array=w703) -> (size(s)=w702:i32)
        n426 = for {
          N: w699 -> [_]
          tunnel: w702 -> [w778]
          tunnel: w669 -> [w777] mode=indexing
          tunnel: [w773] -> w698 mode=indexing
          tunnel: [w764] -> w690 mode=indexing
          tunnel: w630 -> [w758] mode=indexing
          i -> [w766]
          w762 = "WS;" ("string")
          n427 = Quotient & Remainder(x=w766, y=2) -> (x-y*floor(x/y)=w768:i32)  [unwired: 1 out]
          n428 = Equal To 0?(x=w768) -> (x = 0?=w765:bool)
          n429 = for {
            N: w778 -> [_]
            tunnel: w777 -> [w784] mode=indexing
            tunnel: [w782] -> w772 mode=indexing
            tunnel: w765 -> [w781]
            tunnel: [w780] -> w764 mode=indexing
            tunnel: w758 -> [w779] mode=indexing
            n430 = Greater Than 0?(x=w784) -> (x > 0?=w783:bool)
            n431 = case shown="True" w783 {
              tunnel: w784 -> [_ w797]
              tunnel: ["" w804] -> w782
              tunnel: w781 -> [_ w801]
              tunnel: [0 w794] -> w780
              tunnel: w779 -> [_ w787]
              frame False {
              }
              frame True {
                w792 = "WS;" ("string")
                n432 = case shown="False" w787 {
                  tunnel: [w806 w807] -> w791
                  frame False {
                    w806 = 5000  # Max Axis Speed
                  }
                  frame True {
                    n433 = local read "Axes speed \n(µm/s)"() -> (w807:i32)
                  }
                }
                n434 = Divide(x=w797, y=1000) -> (x/y=w799:dbl)
                n435 = case shown="True" w801 {
                  tunnel: w799 -> [w809 w810]
                  tunnel: [w808 w810] -> w800
                  frame False {
                    n436 = Negate(x=w809) -> (-x=w808:dbl)
                  }
                  frame True {
                  }
                }
                n437 = Divide(x=w797, y=w791) -> (x/y=w796:dbl)
                n438 = Multiply(x=w796, y=1000) -> (x*y=w795:dbl)
                n439 = Number To Fractional String(number=w800, width (-)=i16 0, precision (6)=i16 3) -> (F-format string=w788:string)  [unwired: 1 in]
                n440 = local read "X"() -> (w790:string)
                n441 = local read "Y"() -> (w793:string)
                n442 = Round To Nearest(number=w795) -> (nearest integer value=w794:dbl)
                n443 = Concatenate Strings(w790, w792, w793, w792, w790, "PR" ("string"), w788) -> (w804:string)
              }
            }
          }
          n444 = local read "Y Step size in µm"() -> (w776:i32)
          n445 = Divide(x=w776, y=1000) -> (x/y=w771:dbl)
          n446 = Number To Fractional String(number=w771, width (-)=i16 0, precision (6)=i16 3) -> (F-format string=w759:string)  [unwired: 1 in]
          n447 = local read "Y"() -> (w761:string)
          n448 = local read "X"() -> (w763:string)
          n449 = Concatenate Strings(w763, w762, w761, w762, w761, "PR" ("string"), w759) -> (w774:string)
          n450 = Build Array (concatenate)(w772, w774) -> (w773:string[])
        }
        "Commands array" <- w698
        n451 = Index Array(array=w690, index (col)=0 ("disabled index (col)")) -> (element=w692:dbl[])  [unwired: 1 in]
        n452 = Array Size(array=w692) -> (size(s)=w691:i32)
        n453 = for {
          N: w691 -> [w751]
          tunnel: w690 -> [w754] mode=indexing
          tunnel: [w753] -> w634 mode=indexing
          tunnel: [w750] -> w651
          i -> [w752]
          w749 = 5000.0  # Max Axes Speed in µm/s
          n454 = Build Array (concatenate)(w754, w749) -> (w753:dbl[])
          n455 = Equal?(x=w751, y=w752) -> (x = y?=w750:bool)
        }
        "Time array" <- w634
        n456 = Add Array Elements(numeric array=w634) -> (sum=w633:dbl)
        n457 = Quotient & Remainder(x=w633, y=1000.0) -> (floor(x/y)=→"Processi time (sec)":dbl)  [unwired: 1 out]
        n458 = case shown="True" w651 {
          tunnel: ["" "Processing done"] -> w679
          frame False {
          }
          frame True {
          }
        }
      }
    }
    n459 = Get Date/Time In Seconds() -> (seconds since 1Jan1904=w623:timestamp)
    n460 = Format Date/Time String(time format string (%c)="%m/%d/%y -%I:%M %p  ", seconds (now)=w623) -> (date/time string=w622:string)  [unwired: 1 in]
    n461 = Concatenate Strings(w622, w625, "\r") -> (w627:string)
    n462 = invoke on="Log" class="Str" method="Append String"("string"=w627) -> ()  [unwired: 3 in, 4 out]
  }
  n463 = while "Laser control & Stages Control" {
    stop <- w901 stop-if-true
    n464 = event shown="[5] \"EXIT\": Value Change" {
      selector: _ -> [_ _ _ _ _ _ _ _ _ _ _ _]
      dyn-events: _ -> [_ _ _ _ _ _ _ _ _ _ _ _]
      timeout: _ -> [_ _ _ _ _ _ _ _ _ _ _ _]
      tunnel: [_ _ _ _ _ w965 _ _ _ _ _ _] -> w901
      tunnel: [w902 w908 w927 w949 w955 _ _ w996 "Running program..." ("string") w1025 "Opening ESP300 manual" ("StringOut") w1068] -> w898
      event "Energy (%)": Value Change {
        n465 = event-data() -> ()  [unwired: 1 in, 6 out]
        n466 = local read "Energy (%)"() -> (w906:i16)
        n467 = call "IR_Laser_Control.vi"("Action"=T7."Adjust Energy", "Energy (0 - 100)"=w906) -> ()  [unwired: 13 in, 1 out]
        n468 = Number To Decimal String(number=w906, width (-)=i16 3) -> (decimal integer string=w904:string)
        n469 = Concatenate Strings("Energy set to: " ("string"), w904) -> (w902:string)
      }
      event "LAMP": Value Change {
        n470 = event-data() -> ()  [unwired: 1 in, 6 out]
        n471 = local read "LAMP"() -> (w909:bool)
        n472 = case shown="False" w909 {
          tunnel: ["Lamp has been switched off" w914] -> w908
          frame False {
            w911 = FALSE ("Visible")
            n473 = property on="LASER" class="Bool (strict)"("Visible"=w911) -> ()  [unwired: 2 in, 2 out]
            n474 = property on="LAMP" class="Bool (strict)"("BoolText.Text"="LAMP OFF" ("Boolean Text.Text")) -> ()  [unwired: 2 in, 2 out]
            n475 = call "IR_Laser_Control.vi"("Action"=T7."Lamp OFF") -> ()  [unwired: 14 in, 1 out]
            n476 = property on="Capture" class="Bool"("Visible"=w911) -> ()  [unwired: 2 in, 2 out]
          }
          frame True {
            n477 = flat-sequence {
              tunnel: ["Lamp has been switched on"] -> w914
              frame #0 {
                n478 = while {
                  i -> [w919]
                  stop <- w922 stop-if-true
                  n479 = Wait Until Next ms Multiple(millisecond multiple=u32 1000) -> ()  [unwired: 1 out]
                  n480 = Equal?(x=10, y=w919) -> (x = y?=w922:bool)
                  n481 = Subtract(x=10, y=w919) -> (x-y=w917:i32)
                  n482 = Number To Decimal String(number=w917) -> (decimal integer string=w918:string)  [unwired: 1 in]
                  n483 = property on="LAMP" class="Bool (strict)"("BoolText.Text"=w918) -> ()  [unwired: 2 in, 2 out]
                }
                n484 = Wait (ms)(milliseconds to wait=u32 10000) -> ()  [unwired: 1 out]
                n485 = call "IR_Laser_Control.vi"("Action"=T7."Lamp ON") -> ()  [unwired: 14 in, 1 out]
              }
              frame #1 {
                w925 = TRUE ("Visible")
                n486 = property on="Capture" class="Bool"("Visible"=w925) -> ()  [unwired: 2 in, 2 out]
                n487 = property on="LASER" class="Bool (strict)"("Visible"=w925) -> ()  [unwired: 2 in, 2 out]
                n488 = property on="LAMP" class="Bool (strict)"("BoolText.Text"="LAMP ON" ("Boolean Text.Text")) -> ()  [unwired: 2 in, 2 out]
              }
            }
          }
        }
      }
      event "LASER": Value Change {
        n489 = event-data() -> ()  [unwired: 1 in, 6 out]
        n490 = local read "LASER"() -> (w929:bool)
        n491 = case shown="True" w929 {
          tunnel: [w933 w937] -> w928
          tunnel: ["Q-Switch has switched off" w936] -> w927
          frame False {
            w933 = FALSE ("Boolean")
            n492 = property on="LASER" class="Bool (strict)"("BoolText.Text"="LASER OFF" ("Boolean Text.Text"), "Value"=w933) -> ()  [unwired: 2 in, 2 out]
            n493 = call "IR_Alignment_Diode.vi"("AD Action"=enum16{"AD Off", "AD On"}."AD On") -> ()  [unwired: 14 in, 1 out]
            n494 = call "IR_Laser_Control.vi"("Action"=T7."Q-switch OFF") -> ()  [unwired: 14 in, 1 out]
            n495 = property on="Capture" class="Bool"("Visible"=TRUE) -> ()  [unwired: 2 in, 2 out]
            n496 = property on="Laser Operation" class="Bool (strict)"("Blinking"=w933) -> ()  [unwired: 2 in, 2 out]
          }
          frame True {
            n497 = property on="LAMP" class="Bool (strict)"() -> ("BoolText.Text"=w940:string)  [unwired: 2 in, 2 out]
            n498 = Equal?(x=w940, y="LAMP ON") -> (x = y?=w938:bool)
            n499 = case shown="True" w938 {
              tunnel: [FALSE ("Boolean") w946] -> w937
              tunnel: ["Q-Switch has switched off" "Q-Switch has switched on"] -> w936
              frame False {
              }
              frame True {
                w946 = TRUE ("Boolean")
                n500 = call "IR_Alignment_Diode.vi"("AD Action"=enum16{"AD Off", "AD On"}."AD Off") -> ()  [unwired: 14 in, 1 out]
                n501 = property on="Laser Operation" class="Bool (strict)"("Blinking"=w946) -> ()  [unwired: 2 in, 2 out]
                n502 = property on="LASER" class="Bool (strict)"("BoolText.Text"="LASER ON" ("Boolean Text.Text")) -> ()  [unwired: 2 in, 2 out]
                n503 = call "IR_Laser_Control.vi"("Action"=T7."Q-switch ON") -> ()  [unwired: 14 in, 1 out]
                n504 = property on="Capture" class="Bool"("Visible"=FALSE) -> ()  [unwired: 2 in, 2 out]
              }
            }
          }
        }
        "Laser Operation" <- w928
      }
      event "Repetition \nRate": Value Change {
        n505 = event-data() -> ()  [unwired: 1 in, 6 out]
        n506 = local read "Repetition \nRate"() -> (w950:enum16{"1", "2", "5", "10", "20"})
        n507 = call "IR_Laser_Control.vi"("Action"=T7."Change Rep. Rate", "Rep. Rate Divider"=w950) -> ()  [unwired: 13 in, 1 out]
        n508 = Number To Decimal String(number=w950, width (-)=i16 3) -> (decimal integer string=w952:string)
        n509 = Concatenate Strings("Repetition rate set to: " ("string"), w952) -> (w949:string)
      }
      event "TUNE": Value Change {
        n510 = event-data() -> ()  [unwired: 1 in, 6 out]
        n511 = property on="LASER" class="Bool (strict)"() -> ("BoolText.Text"=w962:string)  [unwired: 2 in, 2 out]
        n512 = Equal?(x=w962, y="LASER ON") -> (x = y?=w960:bool)
        n513 = case shown="True" w960 {
          tunnel: [w963 w964] -> w956
          frame False {
            n514 = local read "Wavelength"() -> (w963:dbl)
            n515 = call "IR_Wavelength_Tuning.vi"("Wavelength (nm)"=w963) -> ()  [unwired: 14 in, 1 out]
          }
          frame True {
            n516 = local read "Wavelength"() -> (w964:dbl)
          }
        }
        "Current Wavelength" <- w956
        n517 = Number To Decimal String(number=w956, width (-)=i16 3) -> (decimal integer string=w958:string)
        n518 = Concatenate Strings("Wavelength set to: " ("string"), w958) -> (w955:string)
      }
      event "EXIT": Value Change {
        n519 = event-data() -> ()  [unwired: 1 in, 6 out]
        n520 = flat-sequence {
          tunnel: [w968] -> w965
          frame #0 {
            n521 = dll-call lib="D:/Fabrizio/Labview Projects/IR OPO Controller/Branches/Final version/OPOTEK.dll" fn="OPOTEK_Close"() -> ("error_Code"=→"error_Code 3":i32)  [unwired: 5 in, 2 out]
          }
          frame #1 {
            n522 = local read "Stop Live"() -> (w967:bool)
            n523 = case shown="False" w967 {
              tunnel: [FALSE ("EXIT") "EXIT"] -> w968
              frame False {
                n524 = call "Camera still on error.vi"() -> ()  [unwired: 12 in]
              }
              frame True {
                n525 = Get Date/Time In Seconds() -> (seconds since 1Jan1904=w974:timestamp)
                n526 = Format Date/Time String(time format string (%c)="%d%m%y %I-%M %p ", seconds (now)=w974) -> (date/time string=w976:string)  [unwired: 1 in]
                n527 = control-ref of="This VI"() -> (w979:refnum<vi>)
                n528 = call "IR_Laser_Control.vi"("Action"=T7."Lamp OFF") -> ()  [unwired: 14 in, 1 out]
                n529 = property class="VI"(reference=w979) -> ("Path"=w978:path)  [unwired: 1 in, 2 out]
                n530 = control-ref of="This Application"() -> (w986:refnum<vi>)
                n531 = Strip Path(path=w978) -> (stripped path=w981:path)  [unwired: 1 out]
                n532 = Concatenate Strings(w976, "Log File.txt") -> (w980:string)
                n533 = Build Path(base path=w981, name or relative path=w980) -> (appended path=w973:path)
                n534 = property class="App"(reference=w986) -> ("App.Kind"=w985:T9)  [unwired: 1 in, 2 out]
                n535 = Open/Create/Replace File(file path (use dialog)=w973, operation (0:open)=T8."replace or create") -> (refnum out=w983:refnum<file>, cancelled=w984:bool, error out=w982:errorcluster)  [unwired: 4 in]
                n536 = case shown="False" w984 {
                  tunnel: w983 -> [w991 _]
                  tunnel: w982 -> [w989 _]
                  frame False {
                    n537 = local read "Log"() -> (w990:string)
                    n538 = Write to Text File(file (use dialog)=w991, text=w990, error in=w989) -> (refnum out=w988:refnum<file>, error out=w987:errorcluster)  [unwired: 2 out]
                    n539 = Close File(refnum=w988, error in=w987) -> ()  [unwired: 2 out]
                  }
                  frame True {
                  }
                }
                n540 = case shown="\"Run Time System\"" w985 {
                  frame "Development System", Default {
                  }
                  frame "Run Time System" {
                    n541 = control-ref of="This VI"() -> (w992:refnum<vi>)
                    n542 = Quit LabVIEW() -> ()  [unwired: 1 in]
                    n543 = invoke class="VI" method="FP.Close"(reference=w992) -> ()  [unwired: 2 in, 3 out]
                  }
                }
                n544 = local write "EXIT 3"("EXIT") -> ()
                n545 = local write "EXIT 2"("EXIT") -> ()
                n546 = local write "Exit 4"("EXIT") -> ()
              }
            }
          }
        }
      }
      event "Alignment \ndiode": Value Change {
        n547 = event-data() -> ()  [unwired: 1 in, 6 out]
        n548 = local read "Alignment \ndiode"() -> (w993:bool)
        n549 = case shown="False" w993 {
          frame False {
            n550 = call "IR_Alignment_Diode.vi"("AD Action"=enum16{"AD Off", "AD On"}."AD Off") -> ()  [unwired: 14 in, 1 out]
          }
          frame True {
            n551 = call "IR_Alignment_Diode.vi"("AD Action"=enum16{"AD Off", "AD On"}."AD On") -> ()  [unwired: 14 in, 1 out]
          }
        }
      }
      event "Check \nProgram": Value Change {
        n552 = event-data() -> ()  [unwired: 1 in, 6 out]
        n553 = local read "GPIBport"() -> (w997:i32)
        n554 = Number To Decimal String(number=1) -> (decimal integer string=w1001:string)  [unwired: 1 in]
        n555 = call "IR_OPO_esp_gpib_init_system.vi"("Device In"=w997) -> ("Device Out"=w1002:u8)
        n556 = Concatenate Strings(w1001, "LP") -> (w1005:string)
        n557 = Number To Decimal String(number=w1002) -> (decimal integer string=w1000:string)  [unwired: 1 in]
        n558 = GPIB Write(0:w1000, 1:w1005, 2:i16 3 ("mode (0)")) -> (6:w1004:errorcluster)  [unwired: 2 in, 1 out]
        n559 = while {
          shift-right: [w1013] -> _
          shift-left: w1004 -> [w1015]
          tunnel: w1000 -> [w1014]
          shift-right: [w1011] -> w996
          shift-left: "" -> [w1012]
          stop <- w1007 stop-if-true
          n560 = GPIB Read(0:w1014, 1:255 ("byte count"), 2:i16 2 ("mode (0)"), 3:w1015) -> (5:w1010:string, 7:w1013:errorcluster)  [unwired: 1 in, 1 out]
          n561 = Concatenate Strings(w1012, w1010) -> (w1011:string)
          n562 = Match Pattern(string=w1010, regular expression="END") -> (offset past match=w1008:i32)  [unwired: 1 in, 3 out]
          n563 = Greater Than 0?(x=w1008) -> (x > 0?=w1007:bool)
        }
      }
      event "Run Program": Value Change {
        n564 = event-data() -> ()  [unwired: 1 in, 6 out]
        n565 = local read "GPIBport"() -> (w1018:i32)
        n566 = Number To Decimal String(number=1) -> (decimal integer string=w1021:string)  [unwired: 1 in]
        n567 = Concatenate Strings("EX ", w1021) -> (w1019:string)
        n568 = call "esp_gpib_send_ASCII.vi"("ASCII Cmd"=w1019, "Port In"=w1018) -> ()  [unwired: 5 in, 5 out]
      }
      event "Send \nCommand": Value Change {
        n569 = event-data() -> ()  [unwired: 1 in, 6 out]
        n570 = local read "GPIBport"() -> (w1038:i32)
        n571 = local read "GPIB Mode"() -> (w1024:i16)
        n572 = call "esp_gpib_send_ASCII.vi"("mode (0)"=w1024, "ASCII Cmd"="Type a command", "Port In"=w1038) -> ("Delay Out"=w1027:u16, "error out"=w1028:errorcluster, "Status Out"=w1029:i32, "Port Out"=w1030:i32, "StringOut"=w1026:string)  [unwired: 4 in]
        n573 = Reverse String(1:"Type a command") -> (0:w1036:string)
        n574 = String Subset(string=w1036, offset (0)=0, length (rest)=1 ("length (rest)")) -> (substring=w1033:string)
        n575 = Equal?(x=w1033, y="?") -> (x = y?=w1031:bool)
        n576 = case shown="False" w1031 {
          tunnel: w1030 -> [_ w1044]
          tunnel: w1029 -> [_ w1043]
          tunnel: w1028 -> [_ w1042]
          tunnel: w1027 -> [_ w1041]
          tunnel: [w1039 w1040] -> w1025
          tunnel: w1026 -> [w1039 _]
          frame False {
          }
          frame True {
            n577 = call "esp_gpib_read_ASCII.vi"("Port In"=w1044, "Status In"=w1043, "error in"=w1042, "Delay In"=w1041) -> ("StringOut"=w1040:string)  [unwired: 1 in, 4 out]
          }
        }
      }
      event "Open ESP \nManual": Value Change {
        w1053 = FALSE  # wait until completion? (T)
        n578 = event-data() -> ()  [unwired: 1 in, 6 out]
        n579 = control-ref of="This VI"() -> (w1057:refnum<vi>)
        n580 = property class="VI"(reference=w1057) -> ("Path"=w1056:path)  [unwired: 1 in, 2 out]
        n581 = Strip Path(path=w1056) -> (stripped path=w1055:path)  [unwired: 1 out]
        n582 = Build Path(base path=w1055, name or relative path="NewPort ESP300.PDF") -> (appended path=w1047:path)
        n583 = Path To String(path=w1047) -> (string=w1050:string)
        n584 = Concatenate Strings("cmd  /c \"", w1050, "\"" ("string")) -> (w1045:string)
        n585 = call <vilib>:"System Exec.vi"("run minimized? (F)"=TRUE, "wait until completion? (T)"=w1053, "error in (no error)"="error in (no error)", "command line"=w1045) -> ("error out"=→"error out":errorcluster)  [unwired: 4 in, 3 out]
      }
      event "Capture": Value Change {
        n586 = event-data() -> ()  [unwired: 1 in, 6 out]
        n587 = local read "Y"() -> (w1086:string)
        n588 = local read "X"() -> (w1085:string)
        n589 = local read "GPIB Mode"() -> (w1087:i16)
        n590 = local read "GPIBport"() -> (w1088:i32)
        n591 = flat-sequence {
          tunnel: [w1103] -> w1092
          tunnel: [w1102] -> w1091
          tunnel: [w1101] -> w1090
          tunnel: [w1100] -> w1089
          tunnel: w1088 -> [w1097]
          tunnel: w1087 -> [w1094]
          tunnel: w1086 -> [w1096]
          tunnel: w1085 -> [w1095]
          tunnel: [w1096] -> w1084
          tunnel: [w1095] -> w1083
          tunnel: [w1094] -> w1074
          tunnel: w1092 -> [w1120]
          tunnel: w1091 -> [w1119]
          tunnel: w1090 -> [w1118]
          tunnel: w1089 -> [w1117]
          tunnel: w1084 -> [w1107]
          tunnel: w1083 -> [w1106]
          tunnel: [w1111] -> w1082
          tunnel: [w1110] -> w1081
          tunnel: [w1109] -> w1080
          tunnel: [w1108] -> w1079
          tunnel: [w1107] -> w1077
          tunnel: [w1106] -> w1076
          tunnel: w1074 -> [w1105]
          tunnel: [w1105] -> w1073
          tunnel: w1082 -> [w1121]
          tunnel: w1081 -> [w1122]
          tunnel: w1080 -> [w1123]
          tunnel: w1079 -> [w1125]
          tunnel: [w1128] -> w1078
          tunnel: w1077 -> [w1128]
          tunnel: w1076 -> [w1127]
          tunnel: [w1127] -> w1075
          tunnel: w1073 -> [w1124]
          tunnel: [w1125] -> w1067
          tunnel: [w1124] -> w1066
          tunnel: [w1123] -> w1064
          tunnel: [w1122] -> w1063
          tunnel: [w1121] -> w1062
          tunnel: w1078 -> [w1130]
          tunnel: w1075 -> [w1129]
          tunnel: [w1140] -> w1072
          tunnel: [w1139] -> w1071
          tunnel: [w1138] -> w1070
          tunnel: [w1137] -> w1069
          tunnel: w1067 -> [w1136]
          tunnel: w1066 -> [w1135]
          tunnel: [w1135] -> w1065
          tunnel: w1064 -> [w1134]
          tunnel: w1063 -> [w1133]
          tunnel: w1062 -> [w1132]
          tunnel: [w1131] -> w1061
          tunnel: [w1130] -> w1060
          tunnel: [w1129] -> w1059
          tunnel: w1072 -> [w1155]
          tunnel: w1071 -> [w1154]
          tunnel: w1070 -> [w1153]
          tunnel: w1069 -> [_]
          tunnel: w1065 -> [w1152]
          tunnel: w1061 -> [w1150]
          tunnel: w1060 -> [w1149]
          tunnel: w1059 -> [w1148]
          tunnel: ["Capturing..." ("StringOut")] -> w1068
          frame #0 {
            n592 = Concatenate Strings(w1096, "VA5;" ("string"), w1095, "VA5" ("string")) -> (w1104:string)
            n593 = call "esp_gpib_send_ASCII.vi"("mode (0)"=w1094, "ASCII Cmd"=w1104, "Port In"=w1097) -> ("Delay Out"=w1100:u16, "error out"=w1101:errorcluster, "Status Out"=w1102:i32, "Port Out"=w1103:i32)  [unwired: 4 in, 1 out]
          }
          frame #1 {
            w1114 = "PR" ("string")
            n594 = local read "Laser Y offset"() -> (w1113:string)
            n595 = local read "Laser X offset"() -> (w1112:string)
            n596 = Concatenate Strings(w1107, w1114, w1113, ";" ("string"), w1106, w1114, w1112) -> (w1116:string)
            n597 = call "esp_gpib_send_ASCII.vi"("mode (0)"=w1105, "ASCII Cmd"=w1116, "Delay In"=w1117, "error in"=w1118, "Status In"=w1119, "Port In"=w1120) -> ("Delay Out"=w1108:u16, "error out"=w1109:errorcluster, "Status Out"=w1110:i32, "Port Out"=w1111:i32)  [unwired: 1 in, 1 out]
          }
          frame #2 {
            n598 = Wait (ms)(milliseconds to wait=u32 3000) -> ()  [unwired: 1 out]
          }
          frame #3 {
            w1145 = "VA" ("string")
            n599 = local read "Axes speed \n(µm/s)"() -> (w1144:i32)
            n600 = Divide(x=w1144, y=1000) -> (x/y=w1142:dbl)
            n601 = Number To Fractional String(number=w1142, precision (6)=i16 3) -> (F-format string=w1131:string)  [unwired: 2 in]
            n602 = Concatenate Strings(w1130, w1145, w1131, ";" ("string"), w1129, w1145, w1131) -> (w1147:string)
            n603 = call "esp_gpib_send_ASCII.vi"("mode (0)"=w1135, "ASCII Cmd"=w1147, "Delay In"=w1136, "error in"=w1134, "Status In"=w1133, "Port In"=w1132) -> ("Delay Out"=w1138:u16, "error out"=w1137:errorcluster, "Status Out"=w1139:i32, "Port Out"=w1140:i32)  [unwired: 1 in, 1 out]
          }
          frame #4 {
            n604 = local read "Laser on/off array"() -> (w1157:bool[][])
            n605 = local read "Commands array"() -> (w1159:string[][])
            n606 = local read "Alignment \ndiode"() -> (w1158:bool)
            n607 = local read "Time array"() -> (w1156:dbl[][])
            n608 = call "IR_OPO_Capture.vi"("GPIB Mode"=w1152, "STOP CAPTURE"=FALSE, "Y"=w1149, "Delay"="Delay", "ESP Port"=w1155, "Delay In"=w1153, "Axis Speed"=w1150, "Status In"=w1154, "Commands array"=w1159, "Laser on/off array 2"=w1157, "AD status"=w1158, "X"=w1148, "Time array 2"=w1156) -> ()  [unwired: 3 in]
          }
          frame #5 {
          }
        }
        n609 = case shown="True" FALSE {
          frame False {
          }
          frame True {
            n610 = control-ref of="This VI"() -> (w1162:refnum<vi>)
            n611 = invoke class="VI" method="FP.Close"(reference=w1162) -> ()  [unwired: 2 in, 3 out]
          }
        }
      }
    }
    n612 = Get Date/Time In Seconds() -> (seconds since 1Jan1904=w896:timestamp)
    n613 = Format Date/Time String(time format string (%c)="%m/%d/%y -%I:%M %p  ", seconds (now)=w896) -> (date/time string=w895:string)  [unwired: 1 in]
    n614 = Concatenate Strings(w895, w898, "\r") -> (w900:string)
    n615 = invoke on="Log" class="Str" method="Append String"("string"=w900) -> ()  [unwired: 3 in, 4 out]
  }
  n616 = while "Processing Time Unit" {
    stop <- w1163 stop-if-true
    n617 = event shown="[1] \"Processing time unit\": Value Change" {
      selector: _ -> [_ _]
      dyn-events: _ -> [_ _]
      timeout: _ -> [_ _]
      tunnel: ["EXIT 2" _] -> w1163
      event "EXIT": Value Change {
        n618 = event-data() -> ()  [unwired: 1 in, 3 out]
      }
      event "Processing time unit": Value Change {
        n619 = event-data() -> ()  [unwired: 1 in, 3 out]
        n620 = local read "Processing time unit"() -> (w1167:string)
        n621 = Equal?(x=w1167, y="min") -> (x = y?=w1165:bool)
        n622 = case shown="True" w1165 {
          frame False {
            n623 = local read "Processi time (sec)"() -> (w1168:i32)
            n624 = local write "Process time"(w1168) -> ()
          }
          frame True {
            n625 = local read "Processi time (sec)"() -> (w1170:i32)
            n626 = Quotient & Remainder(x=w1170, y=60) -> (floor(x/y)=w1169:i32)  [unwired: 1 out]
            n627 = local write "Process time"(w1169) -> ()
          }
        }
      }
    }
  }
